vi "backup_imp_test_v9_4.vi"() -> ()   [LabVIEW 2014]
uses:
  <vilib>/eio/EIOPropertyNode/EIOPropertyNode.xnode
  <vilib>/LabVIEW Targets/FPGA/cRIO/shared/nicrio_ModuleControls/nicrio_cRIO-9237_DataRatesRing.ctl
  <vilib>/LabVIEW Targets/FPGA/cRIO/shared/nicrio_ModuleControls/nicrio_cRIO-9237_ExcitationVoltageRing.ctl
  <vilib>/rvi/eio/common/nirviEmuTemplatePropertyGet_errors.vi
  <vilib>/rvi/eio/common/nirviEmuTemplatePropertyGet_noerrors.vi
  <vilib>/rvi/eio/common/nirviEmuTemplatePropertySet_errors.vi
  <vilib>/rvi/eio/common/nirviEmuTemplatePropertySet_noerrors.vi
  <vilib>/eio/EIONode/EIONode.xnode
  <vilib>/rvi/eio/common/nirviEmuTemplateMethod_errors.vi
  <vilib>/rvi/Analysis/measure/butterworth/XNode/niFpgaButterworthFilter.xnode
  <vilib>/rvi/DataTransferAndStorage/Container/XNode/niFpgaContainer.xnode
  <vilib>/rvi/FXPMathLib/FxpSinAndCos/XNode/nifxpmath_SinAndCos.xnode
  <vilib>/rvi/FXPMathLib/FxpSinAndCos/simVIs/DllFxpSinAndCosTemp_sub.vi
  <vilib>/rvi/FXPMathLib/FxpSinAndCos/subVIs/nifxpmath_SinAndCos_SimConfig.ctl
  <vilib>/rvi/interface/RandomDataEmulation/nirviRandomDataFpgaMultiElementTemplate.vi
panel:
  out "omega_y (T) 2":fxp<+/-,36,13>
  out "Dy_d (T) 2":fxp<+/-,36,13>
  out "omega_p (Mavg)":fxp<+/-,36,13>
  out "Dp_d (Mavg)":fxp<+/-,36,13>
  out "omega_p2 (Mavg)":fxp<+/-,36,14>
  out "Dp2_d (Mavg)":fxp<+/-,36,14>
  out "omega_y2 (Mavg)":fxp<+/-,64,27>
  out "Dy2_d (Mavg)":fxp<+/-,36,14>
  in  "mt0_y2":u32
  in  "mt0_p2":u32
  out "Dy_d (Mavg w. f.)":fxp<+/-,36,14>
  out "Dp_d (Mavg w. f.)":fxp<+/-,36,14>
  in  "Dp_d (Mavg) coeff.":i32[](array[numeric])=[946630756, 63555534]
  in  "Dy_d (Mavg) coeff.":i32[](array[numeric])=[946630756, 63555534]
  out "omega_y (Mavg w. f.)":fxp<+/-,36,14>
  in  "omega_y(Mavg) coeff.":i32[](array[numeric])=[946630756, 63555534]
  out "omega_p (Mavg w. f)":fxp<+/-,36,14>
  in  "omega_P(Mavg) coeff.":i32[](array[numeric])=[946630756, 63555534]
  in  "FIFO":i16(ring) items=["Pitch_F+P", "imp ctrl", "Yaw_F+P"]
  out "PID (kHz)":fxp<+/-,20,10>
  in  "Set 6":bool
  in  "Set 5":bool
  in  "Set 4":bool
  in  "Set 3":bool
  in  "Set 2":bool
  in  "Set 1":bool
  out "Dy1_d (T)":fxp<+/-,36,13>
  out "omega_y1 (T)":fxp<+/-,36,13>
  out "Dp1_d (T)":fxp<+/-,36,13>
  out "omega_p1 (T)":fxp<+/-,36,13>
  out "Dy2_d (T)":fxp<+/-,36,13>
  out "Dp2_d (T)":fxp<+/-,36,13>
  out "omega_y2 (T)":fxp<+/-,36,13>
  out "omega_p2 (T)":fxp<+/-,36,13>
  out "mt_omega_y2":u32
  out "mt_omega_p2":u32
  out "rad_y2":fxp<+/-,33,20>
  out "D_y2":fxp<+/-,32,7>
  out "rad_y1":fxp<+/-,33,20>
  out "D_y1":fxp<+/-,32,7>
  out "Encoder Position_y1":i32
  out "Encoder Position_y2":i32
  out "Encoder Position_p2":i32
  out "D_p2":fxp<+/-,32,7>
  out "rad_p2":fxp<+/-,33,20>
  out "D_p1":fxp<+/-,32,7>
  out "rad_p1":fxp<+/-,33,20>
  out "Encoder Position_p1":i32
  in  "Mag. factor_y":fxp<+/-,20,3>
  in  "Mag. encoder_y":bool
  out "omega_y (rad/s)":fxp<+/-,36,13>
  out "Dy_d (mm/s)":fxp<+/-,36,13>
  in  "Vy. Est.":i16(ring) items=["T", "Mavg", "Mavg w. f."]
  out "omega_y1 (Mavg)":fxp<+/-,36,14>
  out "Dy1_d (Mavg)":fxp<+/-,36,14>
  in  "Dy_d_M_avg_Tc (uSec)":i32
  out "Dp1_d (Mavg)":fxp<+/-,36,14>
  out "omega_p1 (Mavg)":fxp<+/-,36,14>
  in  "Dp_d_M_avg_Tc (uSec)":i32
  out "Dp_d (T)":fxp<+/-,36,13>
  out "omega_p (T)":fxp<+/-,36,13>
  in  "Vp. Est.":i16(ring) items=["T", "Mavg", "Mavg w. f."]
  in  "Mag. factor_p":fxp<+/-,20,3>
  in  "Mag. encoder_p":bool
  in  "Belt_out_p":fxp<+/-,7,7>
  in  "Belt_in_p":fxp<+/-,6,6>
  in  "Belt_out_y":fxp<+/-,7,7>
  in  "Belt_in_y":fxp<+/-,6,6>
  out "Fp_dc":fxp<+/-,32,10>
  out "Fy_dc":fxp<+/-,32,10>
  in  "Zero_y":bool
  in  "Zero_p":bool
  in  "mt0_p1":u32
  in  "Encoder reset":bool
  out "fpt_d":fxp<+/-,36,18>
  out "Dp_error_dd":fxp<+/-,36,16>
  out "Dp_error_d":fxp<+/-,33,8>
  in  "Dp_dd coeff.":i32[](array[numeric])=[946630756, 63555534]
  out "Dp_dd":fxp<+/-,36,25>
  out "dFp_PID":fxp<+/-,36,18>
  in  "dFp_PID coeff.":i32[](array[numeric])=[946630756, 63555534]
  out "fpt_i":fxp<+/-,34,18>
  in  "Bv_p":fxp<+/-,22,8>
  in  "Kv_p":fxp<+/-,22,8>
  out "Dp_error":fxp<+/-,22,7>
  out "Dpr_sin":fxp<+/-,22,7>
  in  "Sin offset_p":fxp<+/-,22,7>
  in  "Sin magnitude_p":fxp<+/-,21,6>
  out "Dpr_sin_dd":fxp<+/-,35,20>
  out "Dpr_sin_d":fxp<+/-,33,15>
  out "Sin omega_p":fxp<+/-,34,9>
  in  "Sin wave freq._p (Hz)":fxp<+/-,32,6>
  in  "Dpr_step":fxp<+/-,22,7>
  out "Dpr_for":fxp<+/-,22,7>
  in  "Command_p":i16(ring) items=["Step", "Sine"]
  in  "Ki_p":fxp<+/-,30,9>
  out "Fp_PID":fxp<+/-,36,16>
  in  "fp_tolorance":fxp<+,22,6>
  out "fp_tilde":fxp<+/-,33,10>
  in  "Kd_p":fxp<+/-,30,9>
  in  "Kp_p":fxp<+/-,32,13>
  out "Fr_p":fxp<+/-,32,10>
  in  "S/F coeff_p":fxp<+/-,25,-10>
  in  "S/F coeff_y":fxp<+/-,25,-10>
  out "va_p":fxp<+/-,36,7>
  out "vb_p":fxp<+/-,37,8>
  out "vq_p_F":fxp<+/-,20,5> format="%.57g"
  out "vd_p_F":fxp<+/-,20,5>
  in  "dFp_add":bool
  in  "Stop motor_p":bool
  out "Force_p":fxp<+/-,32,10>
  in  "Strain selection_p":i16(ring) items=["Raw", "Avg.8", "Avg.8 w. filter"]
  out "Strain_p (Avg8 w. f)":fxp<+/-,36,8>
  in  "Strain_p Avg.8 coeff.":i32[](array[numeric])=[946630756, 63555534]
  out "Strain_p (Avg8)":fxp<+/-,36,4>
  out "Raw Strain_p":fxp<+/-,36,4>
  out "Mod6/AI3":fxp<+/-,36,4>
  in  "Strain gage reset_p":bool
  out "Dp_d (mm/s)":fxp<+/-,36,13>
  out "omega_p (rad/s)":fxp<+/-,36,13>
  out "mt_omega_p1":u32
  out "rad_p(NrTheta)":fxp<+/-,33,20>
  out "D_p(mm)":fxp<+/-,32,7>
  out "Encoder Position_p":i32
  in  "Encoder reset_p":bool
  out "Strain_y (Avg8 w. f)":fxp<+/-,36,8>
  in  "Strain_y Avg8 coeff.":i32[](array[numeric])=[-898916953, 1957103773, 3888751]
  out "Dyr_for":fxp<+/-,22,7>
  in  "Command_y":i16(ring) items=["Step", "Sine"]
  out "Strain_y (Avg8)":fxp<+/-,36,4>
  in  "Strain selection_y":i16(ring) items=["Raw", "Avg.8", "Avg.8 w. filter"]
  out "vb_y":fxp<+/-,38,8>
  out "va_y":fxp<+/-,38,8>
  out "fyt_d":fxp<+/-,36,18>
  out "Fr_y":fxp<+/-,32,10>
  in  "Bv_y":fxp<+/-,22,8>
  out "Dy_error_dd":fxp<+/-,36,16>
  out "Dy_error_d":fxp<+/-,33,8>
  in  "Kv_y":fxp<+/-,22,8>
  out "Dy_error":fxp<+/-,22,7>
  out "Dyr_sin_dd":fxp<+/-,35,20>
  out "Dyr_sin_d":fxp<+/-,33,15>
  out "Sin omega_y":fxp<+/-,34,9>
  out "Dyr_sin":fxp<+/-,22,7>
  in  "Sin offset_y":fxp<+/-,22,7>
  in  "Sin magnitude_y":fxp<+/-,21,6>
  out "Time now(s)":fxp<+,52,14>
  in  "Sin wave freq._y (Hz)":fxp<+/-,32,6>
  in  "Dyr_step":fxp<+/-,22,7>
  in  "Drive mode":i16(ring) items=["Backward", "Forward"]
  out "Dy_dd":fxp<+/-,36,25>
  in  "Dy_dd coeff.":i32[](array[numeric])=[946630756, 63555534]
  out "dFy_PID":fxp<+/-,36,18>
  in  "dFy_PID coeff.":i32[](array[numeric])=[946630756, 63555534]
  out "fyt_i":fxp<+/-,36,16>
  out "Fy_PID":fxp<+/-,36,16>
  in  "fy_tolorance":fxp<+,22,6>
  in  "Ki_y":fxp<+/-,30,9>
  in  "Kd_y":fxp<+/-,30,9>
  out "fy_tilde":fxp<+/-,32,10>
  in  "Kp_y":fxp<+/-,32,13>
  out "vq_y_F":fxp<+/-,20,5> format="%.57g"
  out "vd_y_F":fxp<+/-,20,5>
  in  "dFy_add":bool
  in  "Stop motor_y":bool
  out "Dy_d (T)":fxp<+/-,36,13>
  out "omega_y (T)":fxp<+/-,36,13>
  in  "mt0_y1":u32
  out "mt_omega_y1":u32
  out "rad_y(NrTheta)":fxp<+/-,33,20>
  out "D_y(mm)":fxp<+/-,32,7>
  out "Encoder Position_y":i32
  in  "Encoder reset_y":bool
  in  "Ini coe.":bool
  out "Loop rate (kHz)":fxp<+/-,36,7>
  out "Force_y":fxp<+/-,32,10>
  out "Raw Strain_y":fxp<+/-,36,4>
  in  "Strain gage reset_y":bool
  in  "Stop (Strain)":bool
  out "Mod6/AI2":fxp<+/-,36,4>
  in  "Excitation Voltage":T1 items=["2.5 Volts", "3.3 Volts", "5.0 Volts", "10.0 Volts", "External Excitation"]
  in  "Data Rate":T2=1 items=["50.000 kS/s (NI 9237)"=1, "25.000 kS/s (NI 9237)"=2, "16.667 kS/s (NI 9237)"=3, "12.500 kS/s (NI 9237)"=4, "10.000 kS/s (NI 9237)"=5, "8.333 kS/s (NI 9237)"=6, "7.143 kS/s (NI 9237)"=7, "6.250 kS/s (NI 9237)"=8, "5.556 kS/s (NI 9237)"=9, "5.000 kS/s (NI 9237)"=10, "4.545 kS/s (NI 9237)"=11, "4.167 kS/s (NI 9237)"=12, "3.846 kS/s (NI 9237)"=13, "3.571 kS/s (NI 9237)"=14, "3.333 kS/s (NI 9237)"=15, "3.125 kS/s (NI 9237)"=16, "2.941 kS/s (NI 9237)"=17, "2.778 kS/s (NI 9237)"=18, "2.632 kS/s (NI 9237)"=19, "2.500 kS/s (NI 9237)"=20, "2.381 kS/s (NI 9237)"=21, "2.273 kS/s (NI 9237)"=22, "2.174 kS/s (NI 9237)"=23, "2.083 kS/s (NI 9237)"=24, "2.000 kS/s (NI 9237)"=25, "1.923 kS/s (NI 9237)"=26, "1.852 kS/s (NI 9237)"=27, "1.786 kS/s (NI 9237)"=28, "1.724 kS/s (NI 9237)"=29, "1.667 kS/s (NI 9237)"=30, "1.613 kS/s (NI 9237)"=31]
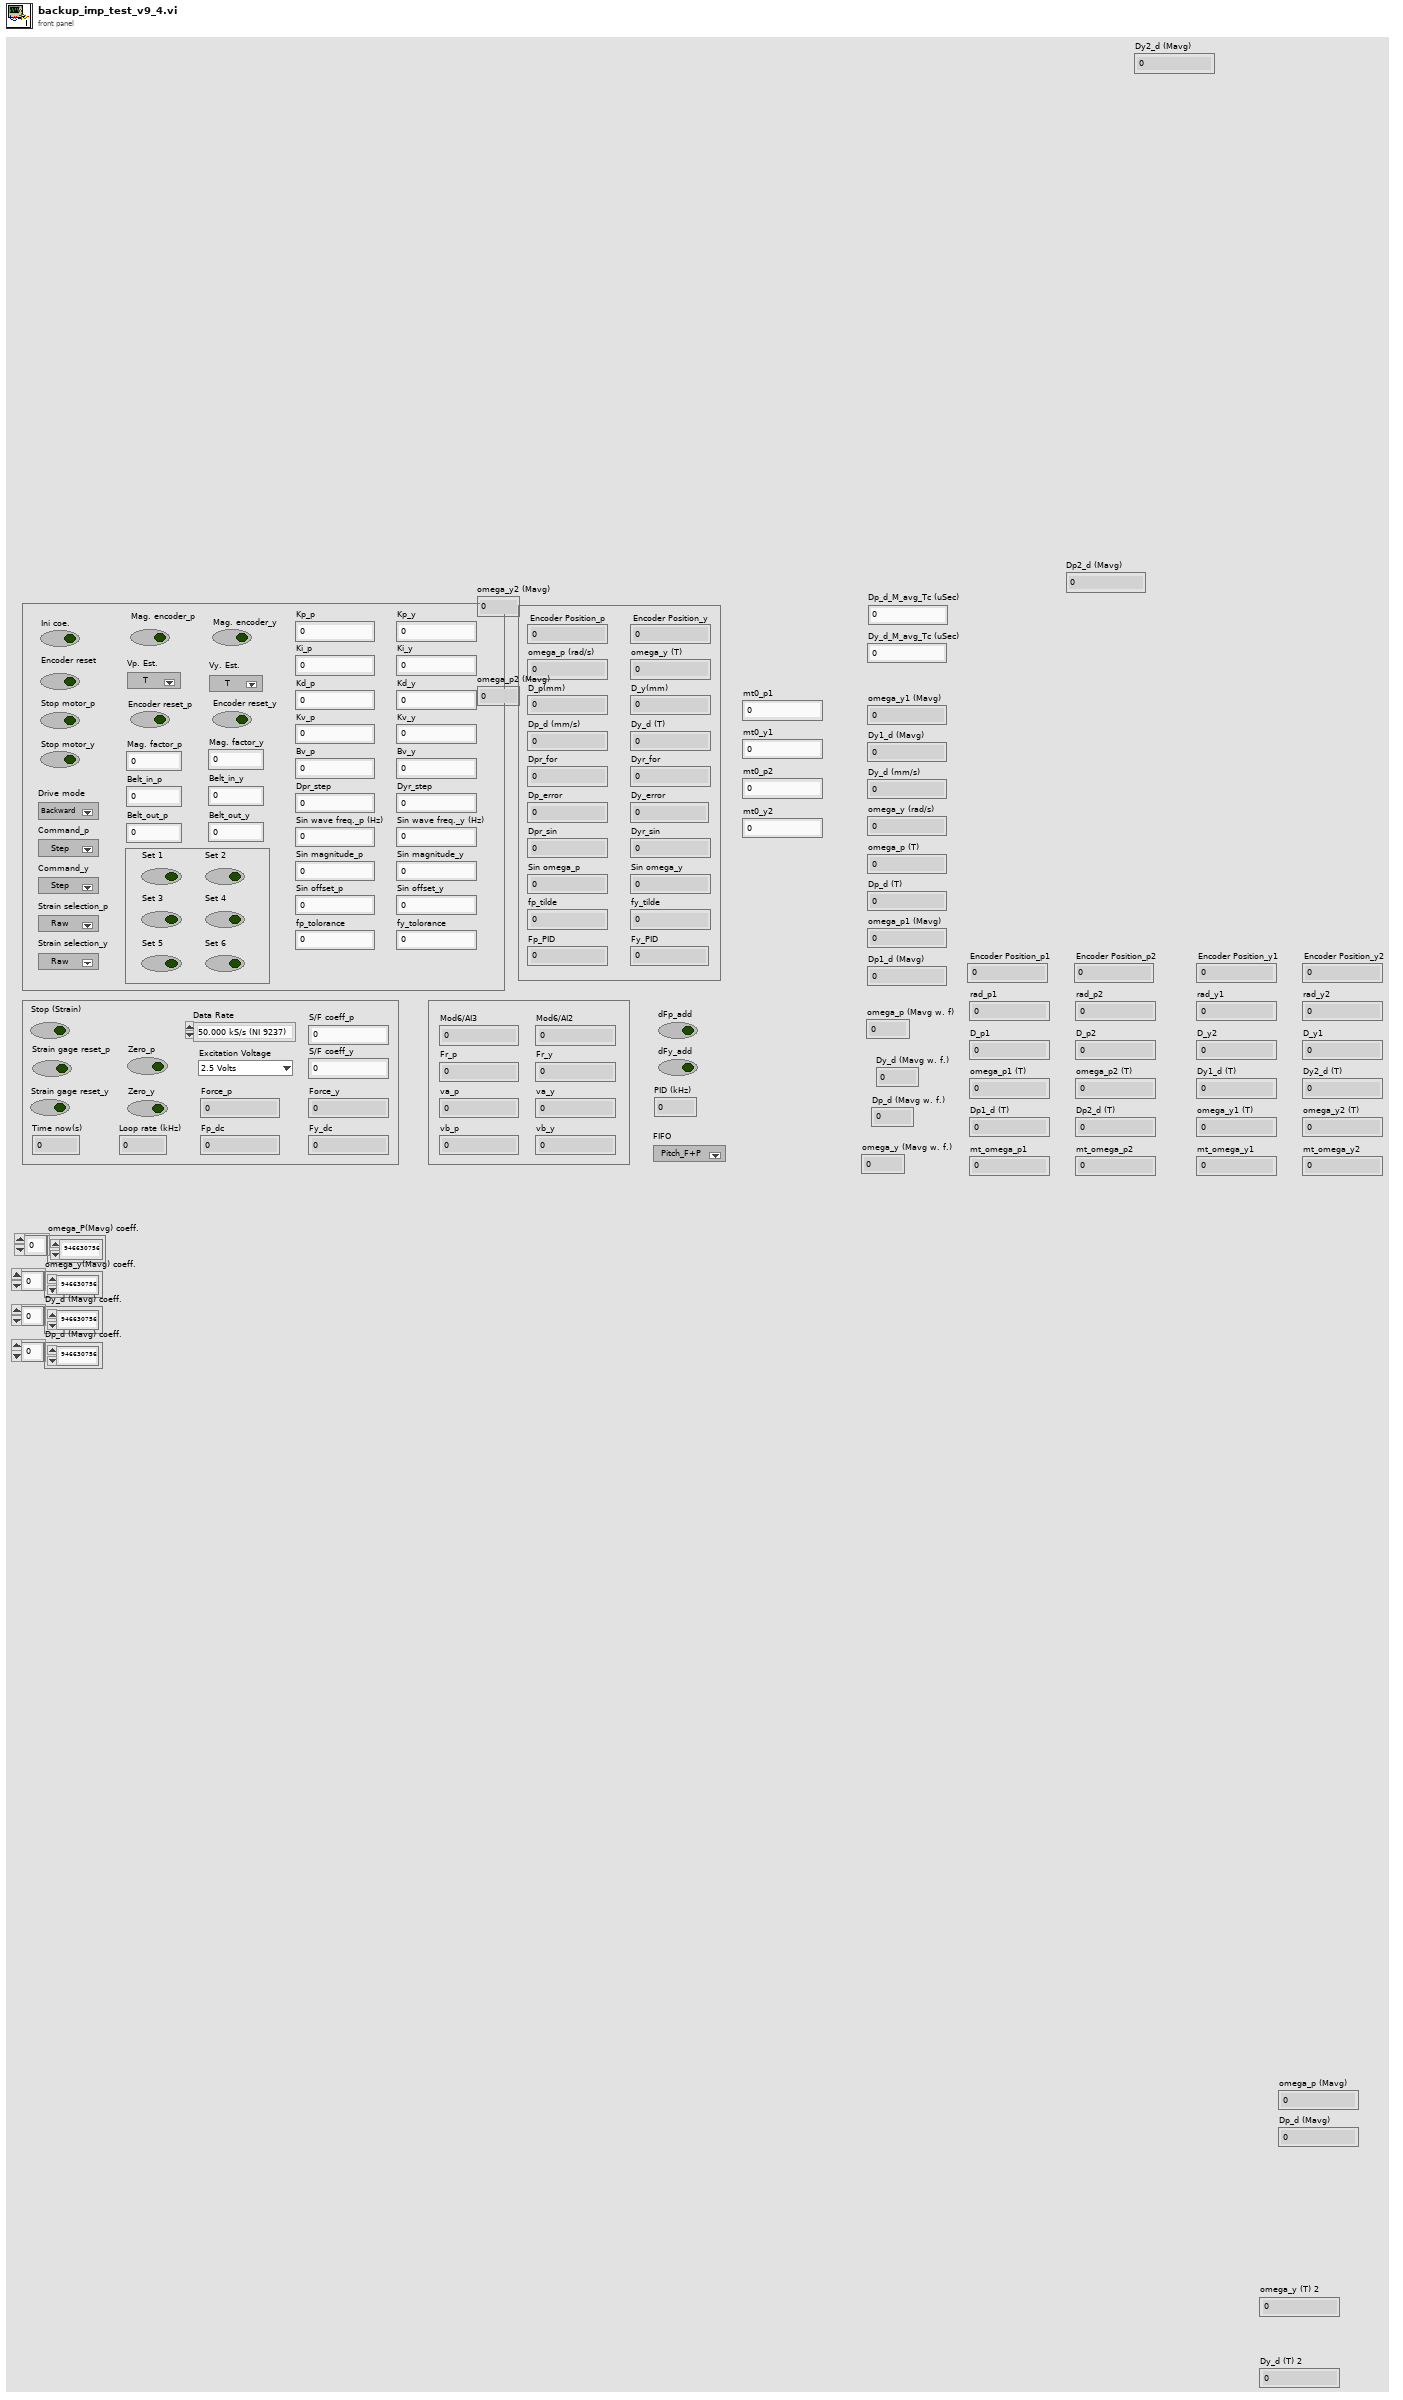
[diagram p1: front panel]
types:
  T1 = typedef "nicrio_cRIO-9237_ExcitationVoltageRing.ctl" = u8
  T2 = typedef "nicrio_cRIO-9237_DataRatesRing.ctl" = u8
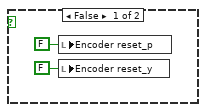
[diagram p12: hidden frame]
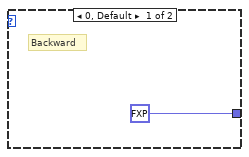
[diagram p13: hidden frame]
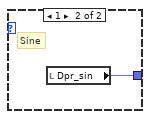
[diagram p14: hidden frame]
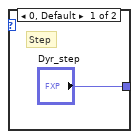
[diagram p15: hidden frame]
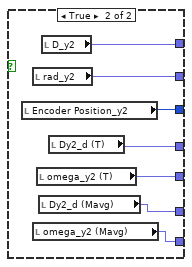
[diagram p16: hidden frame]
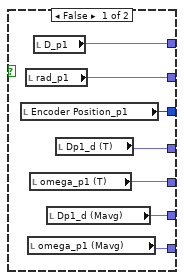
[diagram p17: hidden frame]
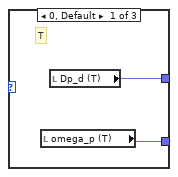
[diagram p18: hidden frame]
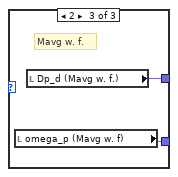
[diagram p19: hidden frame]
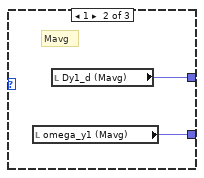
[diagram p20: hidden frame]
diagram:
  w2 = 25
  w5 = i16 25
  w13 = 25
  w16 = 25
  w21 = TRUE ("Half-Bridge Enable")
  # "Encoder 4096ppr\nomega = 61359.2315154/mt\nomega0 = 2*pi/4096 (rad/s)"
  # "Encoder 800ppr\nomega = 314159.265359/mt\nomega0 = 2*pi/800 (rad/s)"
  # "v9\nKp改32/13\nKd改30/9\nKo改30/9"
  # "Resolutuin of Mag. Encoder = 4096*(F_mag)"
  # "use Mavg method to estimate omega or velocity from magnetic encoder"
  # "為什麼要寫兩個迴圈?\nv9後已修正"
  # "Dr_dd ?"
  # "Dr_d ?"
  n1 = xnode "FPGA I/O Property Node"("error in"=errorcluster {"status"=FALSE, "code"=0, "source"=""}, "Data Rate"="Data Rate", "Excitation Voltage"="Excitation Voltage") -> ("error out"=w26:errorcluster)  [unwired: 1 in, 1 out]
  n2 = xnode "FPGA I/O Property Node"("error in"=w26, "Half-Bridge Enable"=w21) -> ("error out"=w19:errorcluster)  [unwired: 1 in, 1 out]
  n3 = xnode "FPGA I/O Property Node"("Half-Bridge Enable"=w21) -> ("error out"=w18:errorcluster)  [unwired: 2 in, 1 out]
  n4 = Merge Errors(w19, w18) -> (w20:errorcluster)
  n5 = xnode "FPGA I/O Node"("error in"=w20, "Mod6/Start"=TRUE) -> ("error out"=w24:errorcluster)  [unwired: 1 in, 1 out]
  n6 = while "AO_p" {
    stop <- FALSE stop-if-true
    n7 = flat-sequence {
      frame #0 {
        n8 = local read "rad_p(NrTheta)"() -> (w41:fxp<+/-,33,20>)
        n9 = local read "vq_p_F"() -> (w42:fxp<+/-,20,5>)
        n10 = local read "vd_p_F"() -> (w44:fxp<+/-,20,5>)
        n11 = Select(t=fxp<+/-,20,5> 0.0, s="Stop motor_p", f=w44) -> (s? t:f=w33:fxp<+/-,20,5>)
        n12 = Select(t=fxp<+,1,1> 0.0, s="Stop motor_p", f=w42) -> (s? t:f=w32:fxp<+/-,20,5>)
        n13 = xnode "High Throughput Sine & Cosine"("x (pi)"=w41) -> ("sin(x)"=w35:fxp<+/-,16,2>, "cos(x)"=w34:fxp<+/-,16,2>)
        n14 = Negate(x=w32) -> (-x=w40:fxp<+/-,21,6>)
        n15 = Multiply(x=w33, y=w35) -> (x*y=w39:fxp<+/-,36,7>)
        n16 = Multiply(x=w33, y=w34) -> (x*y=w37:fxp<+/-,36,7>)
        n17 = Multiply(x=w34, y=w32) -> (x*y=w38:fxp<+/-,36,7>)
        n18 = Multiply(x=w35, y=w40) -> (x*y=w36:fxp<+/-,35,6>)
        n19 = Add(x=w39, y=w38) -> (x+y=→"vb_p":fxp<+/-,37,8>)
        n20 = Add(x=w37, y=w36) -> (x+y=→"va_p":fxp<+/-,36,7>)
      }
      frame #1 {
        n21 = local read "Encoder reset_p"() -> (w77:bool)
        n22 = local read "vb_p"() -> (w78:fxp<+/-,37,8>)
        n23 = local read "va_p"() -> (w79:fxp<+/-,36,7>)
        n24 = Select(t=fxp<+,2,2> 3.0, s=w77, f=w79) -> (s? t:f=w85:fxp<+/-,36,7>)
        n25 = Select(t=fxp<+,1,1> 0.0, s=w77, f=w78) -> (s? t:f=w84:fxp<+/-,37,8>)
        n26 = Multiply(x=w85, y=fxp<+/-,1,0> -0.5) -> (x*y=w80:fxp<+/-,36,6>)
        n27 = Multiply(x=w84, y=fxp<+/-,1,0> -0.5) -> (x*y=w81:fxp<+/-,36,6>)
        n28 = xnode "FPGA I/O Node"("Mod8/AO0"=w80, "Mod8/AO1"=w81) -> ()  [unwired: 2 in, 2 out]
      }
    }
  }
  n29 = while "AO_y" {
    stop <- FALSE stop-if-true
    n30 = flat-sequence {
      frame #0 {
        n31 = local read "rad_y(NrTheta)"() -> (w105:fxp<+/-,33,20>)
        n32 = local read "vd_y_F"() -> (w103:fxp<+/-,20,5>)
        n33 = local read "vq_y_F"() -> (w102:fxp<+/-,20,5>)
        n34 = Select(t=fxp<+/-,20,5> 0.0, s="Stop motor_y", f=w103) -> (s? t:f=w97:fxp<+/-,20,5>)
        n35 = Select(t=fxp<+/-,20,5> 0.0, s="Stop motor_y", f=w102) -> (s? t:f=w96:fxp<+/-,20,5>)
        n36 = xnode "High Throughput Sine & Cosine"("x (pi)"=w105) -> ("sin(x)"=w99:fxp<+/-,17,2>, "cos(x)"=w98:fxp<+/-,17,2>)
        n37 = Negate(x=w96) -> (-x=w95:fxp<+/-,21,6>)
        n38 = Multiply(x=w97, y=w99) -> (x*y=w94:fxp<+/-,37,7>)
        n39 = Multiply(x=w97, y=w98) -> (x*y=w92:fxp<+/-,37,7>)
        n40 = Multiply(x=w98, y=w96) -> (x*y=w93:fxp<+/-,37,7>)
        n41 = Multiply(x=w99, y=w95) -> (x*y=w91:fxp<+/-,36,6>)
        n42 = Add(x=w94, y=w93) -> (x+y=→"vb_y":fxp<+/-,38,8>)
        n43 = Add(x=w92, y=w91) -> (x+y=→"va_y":fxp<+/-,37,7>)
      }
      frame #1 {
        n44 = local read "Encoder reset_y"() -> (w138:bool)
        n45 = local read "va_y"() -> (w137:fxp<+/-,38,8>)
        n46 = local read "vb_y"() -> (w136:fxp<+/-,38,8>)
        n47 = Select(t=fxp<+,2,2> 3.0, s=w138, f=w137) -> (s? t:f=w142:fxp<+/-,38,8>)
        n48 = Select(t=fxp<+,1,1> 0.0, s=w138, f=w136) -> (s? t:f=w141:fxp<+/-,38,8>)
        n49 = Multiply(x=w142, y=fxp<+/-,1,0> -0.5) -> (x*y=w145:fxp<+/-,39,8>)
        n50 = Multiply(x=w141, y=fxp<+/-,1,0> -0.5) -> (x*y=w146:fxp<+/-,37,6>)
        n51 = xnode "FPGA I/O Node"("Mod8/AO2"=w145, "Mod8/AO3"=w146) -> ()  [unwired: 2 in, 2 out]
      }
    }
  }
  n52 = while "Selection" {
    stop <- FALSE stop-if-true
    # "T = Mag. encoder\nF = Motor encoder"
    n53 = case shown="2" "Strain selection_y" {
      tunnel: [w229 w230 w231] -> w182
      frame 0, Default {
        n54 = local read "Raw Strain_y"() -> (w229:fxp<+/-,36,4>)
      }
      frame 1 {
        n55 = local read "Strain_y (Avg8)"() -> (w230:fxp<+/-,36,4>)
      }
      frame 2 {
        n56 = local read "Strain_y (Avg8 w. f)"() -> (w231:fxp<+/-,36,8>)
      }
    }
    n57 = case shown="1" "Vp. Est." {
      tunnel: [w213 w214 w217] -> w165
      tunnel: [w212 w215 w216] -> w166
      frame 0, Default {
        # "T"
        n58 = local read "omega_p (T)"() -> (w213:fxp<+/-,36,13>)
        n59 = local read "Dp_d (T)"() -> (w212:fxp<+/-,36,13>)
      }
      frame 1 {
        # "Mavg"
        n60 = local read "omega_p1 (Mavg)"() -> (w214:fxp<+/-,36,14>)
        n61 = local read "Dp1_d (Mavg)"() -> (w215:fxp<+/-,36,14>)
      }
      frame 2 {
        # "Mavg w. f."
        n62 = local read "omega_p (Mavg w. f)"() -> (w217:fxp<+/-,36,14>)
        n63 = local read "Dp_d (Mavg w. f.)"() -> (w216:fxp<+/-,36,14>)
      }
    }
    "Dp_d (mm/s)" <- w166
    "omega_p (rad/s)" <- w165
    n64 = Divide(x=w182, y="S/F coeff_y") -> (x/y=w175:fxp<+/-,32,10>)
    n65 = case shown="True" "Zero_y" {
      tunnel: w175 -> [_ w225]
      frame False {
      }
      frame True {
        "Fy_dc" <- w225
      }
    }
    n66 = local read "Fy_dc"() -> (w176:fxp<+/-,32,10>)
    n67 = Subtract(x=w175, y=w176) -> (x-y=→"Force_y":fxp<+/-,33,11>)
    n68 = case shown="2" "Strain selection_p" {
      tunnel: [w226 w227 w228] -> w180
      frame 0, Default {
        n69 = local read "Raw Strain_p"() -> (w226:fxp<+/-,36,4>)
      }
      frame 1 {
        n70 = local read "Strain_p (Avg8)"() -> (w227:fxp<+/-,36,4>)
      }
      frame 2 {
        n71 = local read "Strain_p (Avg8 w. f)"() -> (w228:fxp<+/-,36,8>)
      }
    }
    n72 = case shown="0, Default" "Vy. Est." {
      tunnel: [w219 w221 w223] -> w168
      tunnel: [w218 w220 w222] -> w169
      frame 0, Default {
        # "T"
        n73 = local read "omega_y (T)"() -> (w218:fxp<+/-,36,13>)
        n74 = local read "Dy_d (T)"() -> (w219:fxp<+/-,36,13>)
      }
      frame 1 {
        # "Mavg"
        n75 = local read "omega_y1 (Mavg)"() -> (w220:fxp<+/-,36,14>)
        n76 = local read "Dy1_d (Mavg)"() -> (w221:fxp<+/-,36,14>)
      }
      frame 2 {
        # "Mavg w. f."
        n77 = local read "omega_y (Mavg w. f.)"() -> (w222:fxp<+/-,36,14>)
        n78 = local read "Dy_d (Mavg w. f.)"() -> (w223:fxp<+/-,36,14>)
      }
    }
    "Dy_d (mm/s)" <- w168
    "omega_y (rad/s)" <- w169
    n79 = Divide(x=w180, y="S/F coeff_p") -> (x/y=w172:fxp<+/-,32,10>)
    n80 = case shown="True" "Zero_p" {
      tunnel: w172 -> [_ w224]
      frame False {
      }
      frame True {
        "Fp_dc" <- w224
      }
    }
    n81 = local read "Fp_dc"() -> (w170:fxp<+/-,32,10>)
    n82 = Subtract(x=w172, y=w170) -> (x-y=→"Force_p":fxp<+/-,33,11>)
    n83 = case shown="False" "Mag. encoder_y" {
      tunnel: [w190 w196] -> w156
      tunnel: [w189 w197] -> w157
      tunnel: [w188 w195] -> w159
      tunnel: [w186 w194] -> w153
      tunnel: [w187 w193] -> w152
      tunnel: [w185 w192] -> w148
      tunnel: [w184 w191] -> w147
      frame False {
        n84 = local read "Encoder Position_y1"() -> (w188:i32)
        n85 = local read "omega_y1 (Mavg)"() -> (w184:fxp<+/-,36,14>)
        n86 = local read "Dy1_d (Mavg)"() -> (w185:fxp<+/-,36,14>)
        n87 = local read "rad_y1"() -> (w190:fxp<+/-,33,20>)
        n88 = local read "omega_y1 (T)"() -> (w186:fxp<+/-,36,13>)
        n89 = local read "D_y1"() -> (w189:fxp<+/-,32,7>)
        n90 = local read "Dy1_d (T)"() -> (w187:fxp<+/-,36,13>)
      }
      frame True {
        n91 = local read "Encoder Position_y2"() -> (w195:i32)
        n92 = local read "rad_y2"() -> (w196:fxp<+/-,33,20>)
        n93 = local read "omega_y2 (Mavg)"() -> (w191:fxp<+/-,64,27>)
        n94 = local read "omega_y2 (T)"() -> (w194:fxp<+/-,36,13>)
        n95 = local read "Dy2_d (Mavg)"() -> (w192:fxp<+/-,36,14>)
        n96 = local read "D_y2"() -> (w197:fxp<+/-,32,7>)
        n97 = local read "Dy2_d (T)"() -> (w193:fxp<+/-,36,13>)
      }
    }
    "D_y(mm)" <- w157
    "rad_y(NrTheta)" <- w156
    "Encoder Position_y" <- w159
    "Dy_d (T)" <- w152
    "omega_y (T)" <- w153
    "Dy_d (T) 2" <- w148
    "omega_y (T) 2" <- w147
    n98 = case shown="True" "Mag. encoder_p" {
      tunnel: [w204 w211] -> w161
      tunnel: [w203 w210] -> w162
      tunnel: [w202 w209] -> w163
      tunnel: [w200 w208] -> w155
      tunnel: [w201 w207] -> w154
      tunnel: [w199 w205] -> w151
      tunnel: [w198 w206] -> w150
      frame False {
        n99 = local read "Encoder Position_p1"() -> (w202:i32)
        n100 = local read "rad_p1"() -> (w203:fxp<+/-,33,20>)
        n101 = local read "omega_p1 (Mavg)"() -> (w198:fxp<+/-,36,14>)
        n102 = local read "omega_p1 (T)"() -> (w200:fxp<+/-,36,13>)
        n103 = local read "D_p1"() -> (w204:fxp<+/-,32,7>)
        n104 = local read "Dp1_d (Mavg)"() -> (w199:fxp<+/-,36,14>)
        n105 = local read "Dp1_d (T)"() -> (w201:fxp<+/-,36,13>)
      }
      frame True {
        n106 = local read "Encoder Position_p2"() -> (w209:i32)
        n107 = local read "omega_p2 (Mavg)"() -> (w206:fxp<+/-,36,14>)
        n108 = local read "rad_p2"() -> (w210:fxp<+/-,33,20>)
        n109 = local read "D_p2"() -> (w211:fxp<+/-,32,7>)
        n110 = local read "Dp2_d (Mavg)"() -> (w205:fxp<+/-,36,14>)
        n111 = local read "omega_p2 (T)"() -> (w208:fxp<+/-,36,13>)
        n112 = local read "Dp2_d (T)"() -> (w207:fxp<+/-,36,13>)
      }
    }
    "D_p(mm)" <- w161
    "rad_p(NrTheta)" <- w162
    "Encoder Position_p" <- w163
    "Dp_d (T)" <- w154
    "omega_p (T)" <- w155
    "Dp_d (Mavg)" <- w151
    "omega_p (Mavg)" <- w150
  }
  n113 = while "Quadrature drive_y" {
    stop <- FALSE stop-if-true
    n114 = local read "dFy_PID"() -> (w233:fxp<+/-,36,18>)
    n115 = local read "omega_y (rad/s)"() -> (w241:fxp<+/-,36,13>)
    n116 = local read "Fy_PID"() -> (w234:fxp<+/-,36,16>)
    n117 = Select(t=w233, s="dFy_add", f=fxp<+,1,1> 0.0) -> (s? t:f=w237:fxp<+/-,36,18>)
    n118 = call "Oriental_step_motor_PKP225.vi"("F_Threshold"=fxp<+,12,12> 10.0, "dFmr"=w237, "omega"=w241, "Fmr"=w234) -> ("vq_F"=→"vq_y_F":fxp<+/-,20,5>, "vd_F"=→"vd_y_F":fxp<+/-,20,5>)  [unwired: 6 in]
  }
  n119 = while "Encoder_p" {
    shift-right: [w279] -> _
    shift-left: _ -> [w278]
    shift-right: [w280] -> _
    shift-left: _ -> [w277]
    shift-right: [w274] -> _
    shift-left: _ -> [w276]
    shift-right: [w265] -> _
    shift-left: _ -> [w264]
    shift-right: [w266] -> _
    shift-left: _ -> [w267]
    shift-right: [w261] -> _
    shift-left: _ -> [w262]
    stop <- FALSE stop-if-true
    w257 = fxp<+/-,20,-5> 0.00048828125  # L/4096
    w255 = fxp<+/-,16,1> 0.0244140625  # 2*50/4096
    w273 = fxp<+/-,20,-5> 0.002499997615814209  # L/800
    w247 = fxp<+/-,16,1> 0.125  # 2*50/800
    n120 = xnode "FPGA I/O Node"() -> ("Mod7/DIO0"=w282:bool, "Mod7/DIO1"=w281:bool)  [unwired: 2 in, 2 out]
    n121 = xnode "FPGA I/O Node"() -> ("Mod7/DIO4"=w269:bool, "Mod7/DIO5"=w268:bool)  [unwired: 2 in, 2 out]
    n122 = local read "Encoder reset_p"() -> (w263:bool)
    n123 = call "encoder_sub.vi"("A_pre"=w278, "B_pre"=w277, "Encoder Position_pre"=w276, "A input"=w282, "Encoder Position Reset"="Encoder reset_p", "B input"=w281) -> ("A"=w279:bool, "B"=w280:bool, "Encoder Position (Counts)"=w274:i32)  [unwired: 19 in]
    "Encoder Position_p1" <- w274
    n124 = call "encoder_sub.vi"("A_pre"=w264, "B_pre"=w267, "Encoder Position_pre"=w262, "A input"=w269, "Encoder Position Reset"=w263, "B input"=w268) -> ("A"=w265:bool, "B"=w266:bool, "Encoder Position (Counts)"=w261:i32)  [unwired: 19 in]
    "Encoder Position_p2" <- w261
    n125 = local read "Belt_in_p"() -> (w272:fxp<+/-,6,6>)
    n126 = local read "Belt_in_p"() -> (w258:fxp<+/-,6,6>)
    n127 = local read "Belt_out_p"() -> (w270:fxp<+/-,7,7>)
    n128 = To Fixed-Point(number=w261) -> (fixed-point=w243:fxp<+/-,32,32>)  [unwired: 1 in]
    n129 = To Fixed-Point(number=w274) -> (fixed-point=w248:fxp<+/-,32,32>)  [unwired: 1 in]
    n130 = local read "Belt_out_p"() -> (w260:fxp<+/-,7,7>)
    n131 = local read "Mag. factor_p"() -> (w254:fxp<+/-,20,3>)
    n132 = Divide(x=w257, y="Mag. factor_p") -> (x/y=w256:fxp<+/-,41,13>)
    n133 = Multiply(x=w273, y=w272) -> (x*y=w271:fxp<+/-,26,1>)
    n134 = Multiply(x=w256, y=w258) -> (x*y=w259:fxp<+/-,46,18>)
    n135 = Divide(x=w271, y=w270) -> (x/y=w250:fxp<+/-,33,1>)
    n136 = Divide(x=w259, y=w260) -> (x/y=w245:fxp<+/-,53,18>)
    n137 = Divide(x=w255, y=w254) -> (x/y=w242:fxp<+/-,32,1>)
    n138 = Multiply(x=w248, y=w247) -> (x*y=→"rad_p1":fxp<+/-,33,20>)
    n139 = Multiply(x=w245, y=w243) -> (x*y=→"D_p2":fxp<+/-,37,7>)
    n140 = Multiply(x=w243, y=w242) -> (x*y=→"rad_p2":fxp<+/-,33,20>)
    n141 = Multiply(x=w250, y=w248) -> (x*y=→"D_p1":fxp<+/-,32,7>)
  }
  n142 = while "Integral and derivative" {
    shift-right: [w338] -> _
    shift-left: _ -> [w337]
    shift-right: [w330] -> _
    shift-left: _ -> [w329]
    shift-right: [w340] -> _
    shift-left: _ -> [w341]
    shift-right: [w320] -> _
    shift-left: _ -> [w319]
    shift-right: [w306] -> _
    shift-left: _ -> [w309]
    shift-right: [w299] -> _
    shift-left: _ -> [w298]
    shift-right: [w293] -> _
    shift-left: _ -> [w292]
    shift-right: [w288] -> _
    shift-left: _ -> [w289]
    stop <- FALSE stop-if-true
    # "Pitch"
    # "Yaw"
    n143 = local read "Dp_d (mm/s)"() -> (w288:fxp<+/-,36,13>)
    n144 = local read "Dy_d (mm/s)"() -> (w320:fxp<+/-,36,13>)
    n145 = local read "Fp_PID"() -> (w293:fxp<+/-,36,16>)
    n146 = local read "fp_tilde"() -> (w310:fxp<+/-,33,10>)
    n147 = local read "fp_tolorance"() -> (w313:fxp<+,22,6>)
    n148 = local read "fy_tolorance"() -> (w316:fxp<+,22,6>)
    n149 = local read "fy_tilde"() -> (w342:fxp<+/-,32,10>)
    n150 = local read "Fy_PID"() -> (w340:fxp<+/-,36,16>)
    n151 = Subtract(x=w293, y=w292) -> (x-y=w297:fxp<+/-,37,17>)
    n152 = Subtract(x=w288, y=w289) -> (x-y=w290:fxp<+/-,37,14>)
    n153 = Absolute Value(x=w310) -> (abs(x)=w314:fxp<+,33,10>)
    n154 = Absolute Value(x=w342) -> (abs(x)=w344:fxp<+,32,10>)
    n155 = Subtract(x=w340, y=w341) -> (x-y=w328:fxp<+/-,37,17>)
    n156 = Subtract(x=w320, y=w319) -> (x-y=w322:fxp<+/-,36,11>)
    n157 = Greater?(x=w344, y=w316) -> (0:w345:bool)
    n158 = Greater?(x=w314, y=w313) -> (0:w312:bool)
    n159 = Multiply(x=fxp<+,7,10> 1000.0, y=w297) -> (x*y=w295:fxp<+/-,32,18>)
    n160 = Multiply(x=fxp<+,7,10> 1000.0, y=w290) -> (x*y=w286:fxp<+/-,36,21>)
    n161 = local read "Stop motor_y"() -> (w331:bool)
    n162 = local read "Stop motor_p"() -> (w301:bool)
    n163 = Select(t=w342, s=w345, f=fxp<+/-,33,11> 0.0) -> (s? t:f=w338:fxp<+/-,33,11>)
    n164 = Select(t=w310, s=w312, f=fxp<+,1,1> 0.0) -> (s? t:f=w306:fxp<+/-,33,10>)
    n165 = Multiply(x=fxp<+,7,10> 1000.0, y=w322) -> (x*y=w321:fxp<+/-,36,21>)
    n166 = xnode "Butterworth Filter"("input data"=w295, "scaled coefficients"="dFp_PID coeff.") -> ("output data"=→"dFp_PID":fxp<+/-,36,22>)  [unwired: 1 in]
    n167 = xnode "Butterworth Filter"("input data"=w286, "scaled coefficients"="Dp_dd coeff.") -> ("output data"=→"Dp_dd":fxp<+/-,36,25>)  [unwired: 1 in]
    n168 = Multiply(x=fxp<+,7,10> 1000.0, y=w328) -> (x*y=w325:fxp<+/-,32,18>)
    n169 = Add(x=w337, y=w338) -> (x+y=w343:fxp<+/-,34,12>)
    n170 = Multiply(x=w309, y=w306) -> (x*y=w308:fxp<+/-,34,12>)
    n171 = xnode "Butterworth Filter"("input data"=w321, "scaled coefficients"="Dy_dd coeff.") -> ("output data"=→"Dy_dd":fxp<+/-,36,25>)  [unwired: 1 in]
    n172 = Multiply(x=fxp<+/-,30,12> 0.000499725341796875, y=w343) -> (x*y=w336:fxp<+/-,34,10>)
    n173 = Multiply(x=fxp<+/-,30,12> 0.000499725341796875, y=w308) -> (x*y=w305:fxp<+/-,34,10>)
    n174 = xnode "Butterworth Filter"("input data"=w325, "scaled coefficients"="dFy_PID coeff.") -> ("output data"=→"dFy_PID":fxp<+/-,36,22>)  [unwired: 1 in]
    n175 = Select(t=fxp<+,1,1> 0.0, s=w331, f=fxp<+,1,1> 1.0) -> (s? t:f=w334:fxp<+,1,1>)
    n176 = Select(t=fxp<+,1,1> 0.0, s=w301, f=fxp<+,1,1> 1.0) -> (s? t:f=w303:fxp<+,1,1>)
    n177 = Add(x=w336, y=w329) -> (x+y=w335:fxp<+/-,36,16>)
    n178 = Add(x=w305, y=w298) -> (x+y=w304:fxp<+/-,36,16>)
    n179 = Multiply(x=w335, y=w334) -> (x*y=w330:fxp<+/-,34,18>)
    "fyt_i" <- w330
    n180 = Multiply(x=w304, y=w303) -> (x*y=w299:fxp<+/-,34,18>)
    "fpt_i" <- w299
    n181 = call "Wait"("Count(uSec)"=u32 1000) -> ()  [unwired: 1 out]
  }
  n182 = while {
    stop <- FALSE stop-if-true
    n183 = case shown="True" "Set 3" {
      frame False {
      }
      frame True {
        n184 = local write "fp_tolorance"(fxp<+,22,6> 3.0 ("fp_tolorance")) -> ()
        n185 = local write "Kp_p"(fxp<+/-,36,9> 100.0 ("Kp_p")) -> ()
      }
    }
    n186 = case shown="True" "Set 2" {
      frame False {
      }
      frame True {
        n187 = local write "fp_tolorance"(fxp<+,22,6> 1.5 ("fp_tolorance")) -> ()
        n188 = local write "Kp_p"(fxp<+/-,36,9> 50.0 ("Kp_p")) -> ()
      }
    }
    n189 = case shown="True" "Set 1" {
      frame False {
      }
      frame True {
        n190 = local write "fp_tolorance"(fxp<+,22,6> 3.0 ("fp_tolorance")) -> ()
        n191 = local write "Kp_p"(fxp<+/-,36,9> 50.0 ("Kp_p")) -> ()
      }
    }
    n192 = case shown="True" "Set 5" {
      frame False {
      }
      frame True {
        n193 = local write "fp_tolorance"(fxp<+,22,6> 3.0 ("fp_tolorance")) -> ()
        n194 = local write "Kp_p"(fxp<+/-,36,9> 150.0 ("Kp_p")) -> ()
      }
    }
    n195 = case shown="True" "Set 6" {
      frame False {
      }
      frame True {
        n196 = local write "fp_tolorance"(fxp<+,22,6> 1.5 ("fp_tolorance")) -> ()
        n197 = local write "Kp_p"(fxp<+/-,36,9> 150.0 ("Kp_p")) -> ()
      }
    }
    n198 = case shown="True" "Set 4" {
      frame False {
      }
      frame True {
        n199 = local write "fp_tolorance"(fxp<+,22,6> 1.5 ("fp_tolorance")) -> ()
        n200 = local write "Kp_p"(fxp<+/-,36,9> 100.0 ("Kp_p")) -> ()
      }
    }
  }
  n201 = while "Omega_p(T method)" {
    shift-right: [w429] -> _
    shift-left: _ -> [w427]
    shift-right: [w410] -> _
    shift-left: _ -> [w428]
    shift-right: [w425] -> _
    shift-left: _ -> [w426]
    shift-right: [w403] -> _
    shift-left: _ -> [w402]
    shift-right: [w398] -> _
    shift-left: _ -> [w400]
    shift-right: [w406] -> _
    shift-left: _ -> [w405]
    stop <- FALSE stop-if-true
    w417 = fxp<+/-,32,0> 0.3183098859153688  # L/2/pi
    w422 = fxp<+/-,32,0> 0.3183098859153688  # L/2/pi
    n202 = local read "Encoder Position_p1"() -> (w429:i32)
    n203 = local read "Encoder Position_p2"() -> (w403:i32)
    n204 = call "Tick Count4"() -> ("Tick Count(Ticks)"=w404:u32)
    n205 = call "omega_sub_Encoder_800ppr.vi"("mt0"="mt0_p1", "omega_pre"=w428, "ticks_m_pre"=w426, "ticks"=w404, "count_pre"=w427, "count"=w429) -> ("ticks_m"=w425:u32, "mt"=→"mt_omega_p1":u32, "omega"=w410:fxp<+/-,36,13>)  [unwired: 3 in]
    "omega_p1 (T)" <- w410
    n206 = call "omega_sub_Encoder_4096ppr.vi"("mt0"="mt0_p2", "omega_pre"=w400, "ticks_m_pre"=w405, "ticks"=w404, "count_pre"=w402, "count"=w403) -> ("ticks_m"=w406:u32, "mt"=→"mt_omega_p2":u32, "omega"=w398:fxp<+/-,20,9>)  [unwired: 3 in]
    n207 = local read "Mag. factor_p"() -> (w418:fxp<+/-,20,3>)
    n208 = local read "Belt_in_p"() -> (w415:fxp<+/-,6,6>)
    n209 = local read "Belt_out_p"() -> (w414:fxp<+/-,7,7>)
    n210 = Multiply(x=w422, y="Belt_in_p") -> (x*y=w420:fxp<+/-,38,6>)
    n211 = Multiply(x=w417, y=w415) -> (x*y=w416:fxp<+/-,38,6>)
    n212 = Divide(x=w420, y="Belt_out_p") -> (x/y=w411:fxp<+/-,20,1>)
    n213 = Divide(x=w398, y=w418) -> (x/y=w399:fxp<+/-,32,1>)
    "omega_p2 (T)" <- w399
    n214 = Divide(x=w416, y=w414) -> (x/y=w409:fxp<+/-,45,6>)
    n215 = Multiply(x=w409, y=w399) -> (x*y=→"Dp2_d (T)":fxp<+/-,36,13>)
    n216 = Multiply(x=w411, y=w410) -> (x*y=→"Dp1_d (T)":fxp<+/-,36,13>)
  }
  n217 = while "PD position controller_y" {
    stop <- FALSE stop-if-true
    n218 = case shown="0, Default" "Drive mode" {
      tunnel: [fxp<+/-,62,19> 0.0 w435] -> w431
      frame 0, Default {
        # "Backward"
      }
      frame 1 {
        # "Forward"
        n219 = local read "Dy_error_d"() -> (w437:fxp<+/-,33,8>)
        n220 = local read "D_y(mm)"() -> (w442:fxp<+/-,32,7>)
        n221 = local read "Dyr_for"() -> (w434:fxp<+/-,22,7>)
        n222 = Subtract(x=w434, y=w442) -> (x-y=w441:fxp<+/-,33,8>)
        "Dy_error" <- w441
        n223 = Multiply(x=w441, y="Kv_y") -> (x*y=w439:fxp<+/-,54,15>)
        n224 = Multiply(x=w437, y="Bv_y") -> (x*y=w436:fxp<+/-,55,16>)
        n225 = Add(x=w439, y=w436) -> (x+y=w435:fxp<+/-,55,16>)
      }
    }
    "Fr_y" <- w431
  }
  n226 = while "Command type" {
    stop <- FALSE stop-if-true
    n227 = case shown="1" "Command_y" {
      tunnel: ["Dyr_step" w451] -> w446
      frame 0, Default {
        # "Step"
      }
      frame 1 {
        # "Sine"
        n228 = local read "Dyr_sin"() -> (w451:fxp<+/-,22,7>)
      }
    }
    "Dyr_for" <- w446
    n229 = case shown="0, Default" "Command_p" {
      tunnel: ["Dpr_step" w449] -> w444
      frame 0, Default {
        # "Step"
      }
      frame 1 {
        # "Sine"
        n230 = local read "Dpr_sin"() -> (w449:fxp<+/-,22,7>)
      }
    }
    "Dpr_for" <- w444
  }
  n231 = while "Sine wave gene" {
    stop <- FALSE stop-if-true
    w457 = fxp<+,20,3> 6.2831878662109375  # 2*pi
    w489 = fxp<+,20,3> 6.2831878662109375  # 2*pi
    n232 = local read "Time now(s)"() -> (w495:fxp<+,52,14>)
    n233 = local read "Sin wave freq._y (Hz)"() -> (w488:fxp<+/-,32,6>)
    n234 = Multiply(x="Sin wave freq._y (Hz)", y=fxp<+/-,10,3> 2.0) -> (x*y=w496:fxp<+/-,41,9>)
    n235 = local read "Sin magnitude_y"() -> (w486:fxp<+/-,21,6>)
    n236 = local read "Sin magnitude_y"() -> (w479:fxp<+/-,21,6>)
    n237 = local read "Sin omega_y"() -> (w482:fxp<+/-,34,9>)
    n238 = Multiply(x=w496, y=w495) -> (x*y=w494:fxp<+/-,41,19>)
    n239 = Square(x=w482) -> (x^2=w481:fxp<+,34,18>)
    n240 = xnode "High Throughput Sine & Cosine"("x (pi)"=w494) -> ("sin(x)"=w476:fxp<+/-,16,2>, "cos(x)"=w484:fxp<+/-,16,2>)
    n241 = Multiply(x=w489, y=w488) -> (x*y=w487:fxp<+/-,34,9>)
    "Sin omega_y" <- w487
    n242 = Negate(x=w481) -> (-x=w480:fxp<+/-,35,19>)
    n243 = Multiply(x=w487, y=w486) -> (x*y=w485:fxp<+/-,33,15>)
    n244 = Multiply(x=w480, y=w479) -> (x*y=w478:fxp<+/-,34,20>)
    n245 = Multiply(x=w484, y=w485) -> (x*y=→"Dyr_sin_d":fxp<+/-,33,15>)
    n246 = Multiply(x="Sin magnitude_y", y=w476) -> (x*y=w492:fxp<+/-,37,8>)
    n247 = Multiply(x=w476, y=w478) -> (x*y=→"Dyr_sin_dd":fxp<+/-,35,20>)
    n248 = Add(x=w492, y="Sin offset_y") -> (x+y=→"Dyr_sin":fxp<+/-,37,8>)
    n249 = local read "Sin wave freq._p (Hz)"() -> (w453:fxp<+/-,32,6>)
    n250 = local read "Time now(s)"() -> (w471:fxp<+,52,14>)
    n251 = local read "Sin magnitude_p"() -> (w454:fxp<+/-,21,6>)
    n252 = local read "Sin magnitude_p"() -> (w456:fxp<+/-,21,6>)
    n253 = local read "Sin omega_p"() -> (w455:fxp<+/-,34,9>)
    n254 = Multiply(x="Sin wave freq._p (Hz)", y=fxp<+/-,10,3> 2.0) -> (x*y=w475:fxp<+/-,42,9>)
    n255 = Multiply(x=w475, y=w471) -> (x*y=w472:fxp<+/-,41,19>)
    n256 = Square(x=w455) -> (x^2=w467:fxp<+,34,18>)
    n257 = xnode "High Throughput Sine & Cosine"("x (pi)"=w472) -> ("sin(x)"=w458:fxp<+/-,16,2>, "cos(x)"=w463:fxp<+/-,16,2>)
    n258 = Multiply(x=w457, y=w453) -> (x*y=w470:fxp<+/-,34,9>)
    "Sin omega_p" <- w470
    n259 = Negate(x=w467) -> (-x=w466:fxp<+/-,35,19>)
    n260 = Multiply(x=w470, y=w454) -> (x*y=w469:fxp<+/-,33,15>)
    n261 = Multiply(x=w466, y=w456) -> (x*y=w465:fxp<+/-,35,19>)
    n262 = Multiply(x=w463, y=w469) -> (x*y=→"Dpr_sin_d":fxp<+/-,33,15>)
    n263 = Multiply(x=w458, y=w465) -> (x*y=→"Dpr_sin_dd":fxp<+/-,35,20>)
    n264 = Multiply(x="Sin magnitude_p", y=w458) -> (x*y=w461:fxp<+/-,37,8>)
    n265 = Add(x=w461, y="Sin offset_p") -> (x+y=→"Dpr_sin":fxp<+/-,37,8>)
  }
  n266 = while "Time reset" {
    shift-right: [w568] -> _
    shift-left: _ -> [w569]
    shift-right: [w563] -> _
    shift-left: _ -> [w564]
    stop <- FALSE stop-if-true
    n267 = local read "Stop motor_y"() -> (w570:bool)
    n268 = call "Tick Count3"() -> ("Tick Count(uSec)"=w568:u32)
    n269 = Subtract(x=w568, y=w569) -> (x-y=w567:u32)
    n270 = Add(x=w564, y=w567) -> (x+y=w566:u32)
    n271 = Select(t=u32 0, s=w570, f=w566) -> (s? t:f=w563:u32)
    n272 = To Fixed-Point(number=w563) -> (fixed-point=w562:fxp<+,32,32>)  [unwired: 1 in]
    n273 = Multiply(x=fxp<+,20,-18> 1.0000003385357559e-06, y=w562) -> (x*y=→"Time now(s)":fxp<+,52,14>)
  }
  n274 = while "Ini" {
    stop <- FALSE stop-if-true
    n275 = case shown="True" "Ini coe." {
      frame False {
      }
      frame True {
        w578 = T2 20 items=["50.000 kS/s (NI 9237)"=1, "25.000 kS/s (NI 9237)"=2, "16.667 kS/s (NI 9237)"=3, "12.500 kS/s (NI 9237)"=4, "10.000 kS/s (NI 9237)"=5, "8.333 kS/s (NI 9237)"=6, "7.143 kS/s (NI 9237)"=7, "6.250 kS/s (NI 9237)"=8, "5.556 kS/s (NI 9237)"=9, "5.000 kS/s (NI 9237)"=10, "4.545 kS/s (NI 9237)"=11, "4.167 kS/s (NI 9237)"=12, "3.846 kS/s (NI 9237)"=13, "3.571 kS/s (NI 9237)"=14, "3.333 kS/s (NI 9237)"=15, "3.125 kS/s (NI 9237)"=16, "2.941 kS/s (NI 9237)"=17, "2.778 kS/s (NI 9237)"=18, "2.632 kS/s (NI 9237)"=19, "2.500 kS/s (NI 9237)"=20, "2.381 kS/s (NI 9237)"=21, "2.273 kS/s (NI 9237)"=22, "2.174 kS/s (NI 9237)"=23, "2.083 kS/s (NI 9237)"=24, "2.000 kS/s (NI 9237)"=25, "1.923 kS/s (NI 9237)"=26, "1.852 kS/s (NI 9237)"=27, "1.786 kS/s (NI 9237)"=28, "1.724 kS/s (NI 9237)"=29, "1.667 kS/s (NI 9237)"=30, "1.613 kS/s (NI 9237)"=31] ("Data Rate")
        w595 = i16 0 items=["Step", "Sine"] ("Command_p")
        w596 = i16 2 items=["Raw", "Avg.", "Avg. w. filter"] ("Strain selection_p")
        w597 = i16 0 items=["Step", "Sine"] ("Command_y")
        w598 = i16 2 items=["Raw", "Avg.", "Avg. w. filter"] ("Strain selection_y")
        w600 = fxp<+/-,25,-10> 5.851034075021744e-07  # S/F coeff_p
        w599 = fxp<+/-,25,-10> 1.0477961041033268e-06  # S/F coeff_y
        w606 = i16 0 items=["Backward", "Forward"] ("Drive mode")
        n276 = local write "Sin wave freq._y (Hz)"(fxp<+/-,32,6> 1.0 ("Sin wave freq. (Hz)")) -> ()
        n277 = local write "Sin magnitude_y"(fxp<+/-,22,7> 5.0 ("Sin magnitude")) -> ()
        n278 = local write "fy_tolorance"(fxp<+,22,6> 5.0 ("f_tolorance")) -> ()
        n279 = local write "Sin offset_y"(fxp<+/-,38,9> 0.0 ("Sin offset")) -> ()
        n280 = local write "Dyr_step"(fxp<+/-,22,7> 0.0 ("Dr")) -> ()
        n281 = local write "Kp_y"(fxp<+/-,36,9> 30.0 ("Kp")) -> ()
        n282 = local write "Kd_y"(fxp<+/-,36,9> 0.0 ("Kd")) -> ()
        n283 = local write "Kv_y"(fxp<+/-,22,8> 0.0 ("Kv")) -> ()
        n284 = local write "Bv_y"(fxp<+/-,22,8> 0.0 ("Bv")) -> ()
        n285 = local write "Ki_y"(fxp<+/-,36,9> 0.0 ("Ki")) -> ()
        n286 = local write "S/F coeff_p"(w600) -> ()
        n287 = local write "S/F coeff_y"(w599) -> ()
        n288 = local write "Data Rate"(w578) -> ()
        n289 = local write "dFy_add"(FALSE ("dF_add")) -> ()
        n290 = local write "dFp_add"(FALSE ("dFp_add")) -> ()
        n291 = local write "Sin wave freq._p (Hz)"(fxp<+/-,32,6> 1.0 ("Sin wave freq._p (Hz)")) -> ()
        n292 = local write "Sin magnitude_p"(fxp<+/-,21,6> 5.0 ("Sin magnitude_p")) -> ()
        n293 = local write "fp_tolorance"(fxp<+,22,6> 5.0 ("fp_tolorance")) -> ()
        n294 = local write "Sin offset_p"(fxp<+/-,22,7> 0.0 ("Sin offset_p")) -> ()
        n295 = local write "Dpr_step"(fxp<+/-,22,7> 0.0 ("Dpr_step")) -> ()
        n296 = local write "Kp_p"(fxp<+/-,36,9> 30.0 ("Kp_p")) -> ()
        n297 = local write "Kd_p"(fxp<+/-,36,9> 0.0 ("Kd_p")) -> ()
        n298 = local write "Kv_p"(fxp<+/-,22,8> 0.0 ("Kv_p")) -> ()
        n299 = local write "Bv_p"(fxp<+/-,22,8> 0.0 ("Bv_p")) -> ()
        n300 = local write "Ki_p"(fxp<+/-,36,9> 0.0 ("Ki_p")) -> ()
        n301 = local write "Strain selection_p"(w596) -> ()
        n302 = local write "Strain selection_y"(w598) -> ()
        n303 = local write "Command_p"(w595) -> ()
        n304 = local write "Command_y"(w597) -> ()
        n305 = local write "Drive mode"(w606) -> ()
        n306 = local write "Dp_d_M_avg_Tc (uSec)"(u32 1000 ("D_d_M_avg_Tc (uSec)")) -> ()
        n307 = local write "Dy_d_M_avg_Tc (uSec)"(1000 ("Dy_d_M_avg_Tc (uSec)")) -> ()
        n308 = local write "Belt_out_p"(fxp<+/-,7,7> 36.0 ("Belt_op")) -> ()
        n309 = local write "Belt_out_y"(fxp<+/-,7,7> 22.0 ("Belt_oy")) -> ()
        n310 = local write "Belt_in_p"(fxp<+/-,6,6> 14.0 ("Belt_mp")) -> ()
        n311 = local write "Belt_in_y"(fxp<+/-,6,6> 16.0 ("Belt_my")) -> ()
        n312 = local write "mt0_p1"(u32 40000000 ("mt0_p1")) -> ()
        n313 = local write "mt0_p2"(u32 40000000 ("mt0_p2")) -> ()
        n314 = local write "mt0_y1"(u32 40000000 ("mt0_y1")) -> ()
        n315 = local write "mt0_y2"(u32 40000000 ("mt0_y2")) -> ()
      }
    }
  }
  n316 = while "FIFO" {
    stop <- FALSE stop-if-true
    n317 = flat-sequence {
      frame #0 {
        n318 = call "Loop Timer"("Count(uSec)"=u32 1000) -> ()  [unwired: 1 out]
      }
      frame #1 {
        n319 = case shown="2" "FIFO" {
          tunnel: [w649 w665 w681] -> w633
          tunnel: [w648 w664 w680] -> w632
          tunnel: [w647 w663 w679] -> w631
          tunnel: [w646 w662 w678] -> w630
          tunnel: [w643 w661 w675] -> w628
          tunnel: [w644 w660 w676] -> w627
          tunnel: [w645 w659 w677] -> w626
          tunnel: [w641 w658 w673] -> w625
          tunnel: [w640 w657 w672] -> w624
          tunnel: [w639 w656 w671] -> w623
          tunnel: [w638 w655 w670] -> w622
          tunnel: [w637 w654 w669] -> w621
          tunnel: [w636 w653 w668] -> w620
          tunnel: [w635 w652 w667] -> w619
          tunnel: [w634 fxp<+,1,1> 0.0 ("element") w666] -> w618
          tunnel: [w642 fxp<+,1,1> 0.0 w674] -> w616
          frame 0 {
            # "Pitch"
            n320 = local read "omega_p (Mavg w. f)"() -> (w635:fxp<+/-,36,14>)
            n321 = local read "omega_p1 (Mavg)"() -> (w643:fxp<+/-,36,14>)
            n322 = local read "Dp1_d (Mavg)"() -> (w634:fxp<+/-,36,14>)
            n323 = local read "Encoder Position_p1"() -> (w649:i32)
            n324 = local read "Encoder Position_p2"() -> (w648:i32)
            n325 = local read "D_p1"() -> (w647:fxp<+/-,32,7>)
            n326 = local read "D_p2"() -> (w646:fxp<+/-,32,7>)
            n327 = local read "omega_p1 (T)"() -> (w645:fxp<+/-,36,13>)
            n328 = local read "omega_p2 (T)"() -> (w644:fxp<+/-,36,13>)
            n329 = local read "rad_p1"() -> (w642:fxp<+/-,33,20>)
            n330 = local read "rad_p2"() -> (w641:fxp<+/-,33,20>)
            n331 = local read "Force_p"() -> (w640:fxp<+/-,32,10>)
            n332 = local read "Raw Strain_p"() -> (w639:fxp<+/-,36,4>)
            n333 = local read "Strain_p (Avg8)"() -> (w638:fxp<+/-,36,4>)
            n334 = local read "Strain_p (Avg8 w. f)"() -> (w637:fxp<+/-,36,8>)
            n335 = local read "Dp_d (mm/s)"() -> (w636:fxp<+/-,36,13>)
          }
          frame 1, Default {
            # "imp ctrl"
            n336 = local read "D_y(mm)"() -> (w665:fxp<+/-,32,7>)
            n337 = local read "Raw Strain_y"() -> (w664:fxp<+/-,36,4>)
            n338 = local read "Strain_y (Avg8)"() -> (w663:fxp<+/-,36,4>)
            n339 = local read "Strain_y (Avg8 w. f)"() -> (w662:fxp<+/-,36,8>)
            n340 = local read "Force_y"() -> (w659:fxp<+/-,32,10>)
            n341 = local read "Dy_d (T)"() -> (w660:fxp<+/-,36,13>)
            n342 = local read "Fy_dc"() -> (w661:fxp<+/-,32,10>)
            n343 = local read "D_p(mm)"() -> (w658:fxp<+/-,32,7>)
            n344 = local read "Raw Strain_p"() -> (w657:fxp<+/-,36,4>)
            n345 = local read "Strain_p (Avg8)"() -> (w656:fxp<+/-,36,4>)
            n346 = local read "Strain_p (Avg8 w. f)"() -> (w655:fxp<+/-,36,8>)
            n347 = local read "Force_p"() -> (w654:fxp<+/-,32,10>)
            n348 = local read "Dp_d (mm/s)"() -> (w653:fxp<+/-,36,13>)
            n349 = local read "Fp_dc"() -> (w652:fxp<+/-,32,10>)
          }
          frame 2 {
            # "Yaw"
            n350 = local read "omega_y (Mavg w. f.)"() -> (w667:fxp<+/-,36,14>)
            n351 = local read "omega_y1 (Mavg)"() -> (w675:fxp<+/-,36,14>)
            n352 = local read "Dy1_d (Mavg)"() -> (w666:fxp<+/-,36,14>)
            n353 = local read "Encoder Position_y1"() -> (w681:i32)
            n354 = local read "Encoder Position_y2"() -> (w680:i32)
            n355 = local read "D_y1"() -> (w679:fxp<+/-,32,7>)
            n356 = local read "D_y2"() -> (w678:fxp<+/-,32,7>)
            n357 = local read "omega_y1 (T)"() -> (w677:fxp<+/-,36,13>)
            n358 = local read "omega_y2 (T)"() -> (w676:fxp<+/-,36,13>)
            n359 = local read "rad_y1"() -> (w674:fxp<+/-,33,20>)
            n360 = local read "rad_y2"() -> (w673:fxp<+/-,33,20>)
            n361 = local read "Force_y"() -> (w672:fxp<+/-,32,10>)
            n362 = local read "Raw Strain_y"() -> (w671:fxp<+/-,36,4>)
            n363 = local read "Strain_y (Avg8)"() -> (w670:fxp<+/-,36,4>)
            n364 = local read "Strain_y (Avg8 w. f)"() -> (w669:fxp<+/-,36,8>)
            n365 = local read "Dy_d (mm/s)"() -> (w668:fxp<+/-,36,13>)
          }
        }
        n366 = Build Array(w633, w632, w631, w630, w626, w627, w628, w616, w625, w624, w623, w622, w621, w620, w619, w618) -> (w617:fxp<+/-,64,32>[])
        n367 = xnode ("FIFO Write")("Element"=w617, "Timeout"=0) -> ()  [unwired: 1 in, 2 out]
      }
    }
  }
  n368 = while "PID force controller_y" {
    stop <- FALSE stop-if-true
    n369 = local read "Force_y"() -> (w683:fxp<+/-,32,10>)
    n370 = local read "fyt_d"() -> (w692:fxp<+/-,36,18>)
    n371 = local read "Fr_y"() -> (w684:fxp<+/-,32,10>)
    n372 = Subtract(x=w684, y=w683) -> (x-y=w682:fxp<+/-,33,11>)
    "fy_tilde" <- w682
    n373 = Absolute Value(x=w682) -> (abs(x)=w699:fxp<+,32,10>)
    n374 = local read "fyt_i"() -> (w688:fxp<+/-,36,16>)
    n375 = Multiply(x="Kp_y", y=w682) -> (x*y=w690:fxp<+/-,64,23>)
    n376 = Multiply(x="Kd_y", y=w692) -> (x*y=w691:fxp<+/-,64,27>)
    n377 = Multiply(x="Ki_y", y=w688) -> (x*y=w686:fxp<+/-,64,25>)
    n378 = Add(x=w690, y=w691) -> (x+y=w687:fxp<+/-,64,28>)
    n379 = Greater?(x=w699, y="fy_tolorance") -> (0:w697:bool)
    n380 = Add(x=w687, y=w686) -> (x+y=w685:fxp<+/-,36,16>)
    n381 = Select(t=w685, s=w697, f=fxp<+/-,51,14> 0.0) -> (s? t:f=→"Fy_PID":fxp<+/-,53,16>)
  }
  n382 = for {
    N: w2 -> [_]
    tunnel: [w702] -> w4 mode=indexing
    tunnel: [w701] -> w3 mode=indexing
    tunnel: [w701] -> w1
    n383 = local read "Dy_d_M_avg_Tc (uSec)"() -> (w701:i32)
    n384 = local read "Encoder Position_p2"() -> (w702:i32)
    n385 = call "Wait5"("Count(uSec)"=w701) -> ()  [unwired: 1 out]
  }
  n386 = while {
    tunnel: w24 -> [w747]
    tunnel: [w721] -> w17
    shift-right: [w745] -> _
    shift-left: _ -> [w746]
    shift-right: [w741] -> _
    shift-left: _ -> [w742]
    shift-right: [w736] -> _
    shift-left: _ -> [w735]
    shift-right: [w735] -> _
    shift-left: _ -> [w734]
    shift-right: [w734] -> _
    shift-left: _ -> [w733]
    shift-right: [w733] -> _
    shift-left: _ -> [w732]
    shift-right: [w732] -> _
    shift-left: _ -> [w731]
    shift-right: [w731] -> _
    shift-left: _ -> [w730]
    shift-right: [w730] -> _
    shift-left: _ -> [w729]
    tunnel: w24 -> [w725]
    shift-right: [w718] -> _
    shift-left: _ -> [w719]
    shift-right: [w714] -> _
    shift-left: _ -> [w713]
    shift-right: [w713] -> _
    shift-left: _ -> [w712]
    shift-right: [w712] -> _
    shift-left: _ -> [w711]
    shift-right: [w711] -> _
    shift-left: _ -> [w710]
    shift-right: [w710] -> _
    shift-left: _ -> [w709]
    shift-right: [w709] -> _
    shift-left: _ -> [w708]
    shift-right: [w708] -> _
    shift-left: _ -> [w707]
    stop <- w722 stop-if-true
    w716 = fxp<+,20,2> 2.115001678466797  # Gage Factor
    n387 = xnode "FPGA I/O Node"("error in"=w747) -> ("error out"=w721:errorcluster, "Mod6/AI2"=w743:fxp<+/-,24,-4>)  [unwired: 1 in, 1 out]
    n388 = xnode "FPGA I/O Node"("error in"=w725) -> ("error out"=w723:errorcluster, "Mod6/AI3"=w717:fxp<+/-,24,-4>)  [unwired: 1 in, 1 out]
    n389 = Or(x=w721, y="Stop (Strain)") -> (x .or. y?=w724:bool)
    n390 = Select(t=w717, s="Strain gage reset_p", f=w719) -> (s? t:f=w718:fxp<+/-,24,-4>)
    n391 = Select(t=w743, s="Strain gage reset_y", f=w746) -> (s? t:f=w745:fxp<+/-,24,-4>)
    n392 = Or(x=w724, y=w723) -> (x .or. y?=w722:bool)
    n393 = Subtract(x=w717, y=w718) -> (x-y=w715:fxp<+/-,30,-3>)
    "Mod6/AI3" <- w715
    n394 = Subtract(x=w743, y=w745) -> (x-y=w744:fxp<+/-,30,-3>)
    "Mod6/AI2" <- w744
    n395 = Multiply(x=w716, y=w744) -> (x*y=w736:fxp<+/-,41,6>)
    "Raw Strain_y" <- w736
    n396 = Multiply(x=w716, y=w715) -> (x*y=w714:fxp<+/-,50,-1>)
    "Raw Strain_p" <- w714
    n397 = call "average_v2.vi"("Numeric 8"=w707, "Numeric"=w714, "Numeric 7"=w708, "Numeric 2"=w713, "Numeric 6"=w709, "Numeric 5"=w710, "Numeric 4"=w711, "Numeric 3"=w712) -> ("Mean (8pt)"=w706:fxp<+/-,32,4>)  [unwired: 1 in, 2 out]
    "Strain_p (Avg8)" <- w706
    n398 = call "average_v2.vi"("Numeric 8"=w729, "Numeric"=w736, "Numeric 7"=w730, "Numeric 2"=w735, "Numeric 6"=w731, "Numeric 5"=w732, "Numeric 4"=w733, "Numeric 3"=w734) -> ("Mean (8pt)"=w728:fxp<+/-,32,4>)  [unwired: 1 in, 2 out]
    "Strain_y (Avg8)" <- w728
    n399 = call "Tick Count"() -> ("Tick Count(uSec)"=w741:u32)
    n400 = xnode "Butterworth Filter"("input data"=w706, "scaled coefficients"="Strain_p Avg.8 coeff.") -> ("output data"=→"Strain_p (Avg8 w. f)":fxp<+/-,36,8>)  [unwired: 1 in]
    n401 = xnode "Butterworth Filter"("input data"=w728, "scaled coefficients"="Strain_y Avg8 coeff.") -> ("output data"=→"Strain_y (Avg8 w. f)":fxp<+/-,32,4>)  [unwired: 1 in]
    n402 = Subtract(x=w741, y=w742) -> (x-y=w739:fxp<+/-,32,16>)
    n403 = Divide(x=fxp<+,7,10> 1000.0, y=w739) -> (x/y=→"Loop rate (kHz)":fxp<+/-,40,27>)
  }
  n404 = for {
    N: w5 -> [_]
    tunnel: [w766] -> w8 mode=indexing
    tunnel: [w765] -> w7 mode=indexing
    tunnel: [w764] -> w6
    n405 = local read "Dy_d_M_avg_Tc (uSec)"() -> (w764:i32)
    n406 = local read "Encoder Position_y2"() -> (w766:i32)
    n407 = call "Wait4"("Count(uSec)"=w764) -> ("Tick Count(uSec)"=w765:u32)
  }
  n408 = for {
    N: w13 -> [_]
    tunnel: [w769] -> w12 mode=indexing
    tunnel: [w768] -> w11 mode=indexing
    tunnel: ["Dy_d_M_avg_Tc (uSec)"] -> w10
    n409 = local read "Encoder Position_y1"() -> (w768:i32)
    n410 = call "Wait3"("Count(uSec)"="Dy_d_M_avg_Tc (uSec)") -> ("Tick Count(uSec)"=w769:u32)
  }
  n411 = for {
    N: w16 -> [_]
    tunnel: ["Dp_d_M_avg_Tc (uSec)"] -> w9
    tunnel: [w771] -> w15 mode=indexing
    tunnel: [w770] -> w14 mode=indexing
    n412 = local read "Encoder Position_p1"() -> (w770:i32)
    n413 = call "Wait2"("Count(uSec)"="Dp_d_M_avg_Tc (uSec)") -> ("Tick Count(uSec)"=w771:u32)
  }
  n414 = while "Omega_p2 (Mavg)" {
    shift-right: _ -> [_]
    shift-left: w4 -> [w796]
    shift-right: _ -> [_]
    shift-left: w3 -> [w794]
    shift-right: [w777] -> _
    shift-left: _ -> [w773]
    tunnel: w2 -> [w792]
    tunnel: w1 -> [w797]
    stop <- FALSE stop-if-true
    w778 = fxp<+/-,27,3> 3.1415926814079285  # pi
    w784 = fxp<+,32,0> 0.1953125  # 800/4096
    w789 = fxp<+/-,32,0> 0.3183098859153688  # L/2/pi
    n415 = call "Tick Count9"() -> ("Tick Count(uSec)"=w791:u32)
    n416 = Index Array(array=w794, index=0) -> (element=w793:i32)
    n417 = Index Array(array=w796, index=0) -> (element=w795:i32)
    n418 = Multiply(x=w792, y=w797) -> (x*y=w800:i32)
    n419 = Add(x=w800, y=w793) -> (x+y=w799:i32)
    n420 = Greater Or Equal?(x=w791, y=w799) -> (x >= y?=w798:bool)
    n421 = case shown="True" w798 {
      tunnel: w796 -> [w804 w818]
      tunnel: w795 -> [_ w810]
      tunnel: w794 -> [w805 w819]
      tunnel: w793 -> [_ w820]
      tunnel: w792 -> [_ w817]
      tunnel: w791 -> [_ w821]
      tunnel: [w804 w808] -> _
      tunnel: [w805 w807] -> _
      tunnel: [w803 w806] -> w777
      tunnel: w773 -> [w803 _]
      frame False {
      }
      frame True {
        n422 = local read "Encoder Position_p2"() -> (w809:i32)
        n423 = Subtract(x=w821, y=w820) -> (x-y=w822:u32)
        n424 = Insert Into Array(array=w819) -> (w824:i32[])  [unwired: 2 in]
        n425 = Subtract(x=w809, y=w810) -> (x-y=w814:i32)
        n426 = Insert Into Array(array=w818, index=w817, new element=w809) -> (w825:i32[])
        n427 = To Fixed-Point(number=w822) -> (fixed-point=w811:fxp<+,32,32>)  [unwired: 1 in]
        n428 = Multiply(x=w814, y=2500) -> (x*y=w815:i32)
        n429 = To Fixed-Point(number=w815) -> (fixed-point=w816:fxp<+/-,32,32>)  [unwired: 1 in]
        n430 = Delete From Array(array=w824, length=1, index=0) -> (array with subset deleted=w807:i32[])  [unwired: 1 out]
        n431 = Delete From Array(array=w825, length=1, index=0) -> (array with subset deleted=w808:i32[])  [unwired: 1 out]
        n432 = Divide(x=w816, y=w811) -> (x/y=w806:fxp<+/-,56,22>)
      }
    }
    n433 = local read "Mag. factor_p"() -> (w783:fxp<+/-,20,3>)
    n434 = local read "Mag. encoder_y"() -> (w781:bool)
    n435 = local read "Belt_in_p"() -> (w786:fxp<+/-,6,6>)
    n436 = local read "Belt_out_p"() -> (w785:fxp<+/-,7,7>)
    n437 = Divide(x=w784, y=w783) -> (x/y=w782:fxp<+/-,32,1>)
    n438 = Multiply(x=w778, y=w777) -> (x*y=w780:fxp<+/-,64,25>)
    n439 = Select(t=w782, s=w781, f=fxp<+/-,2,2> 1.0) -> (s? t:f=w776:fxp<+/-,33,2>)
    n440 = Multiply(x=w789, y=w786) -> (x*y=w790:fxp<+/-,38,6>)
    n441 = Multiply(x=w776, y=w780) -> (x*y=→"omega_p2 (Mavg)":fxp<+/-,64,27>)
    n442 = Divide(x=w790, y=w785) -> (x/y=w788:fxp<+/-,45,6>)
    n443 = Multiply(x=w788) -> (x*y=→"Dp2_d (Mavg)":fxp<+/-,64,10>)  [unwired: 1 in]
  }
  n444 = while "Omega_y1 (Mavg)" {
    tunnel: w13 -> [w851]
    shift-right: [w849] -> _
    shift-left: w12 -> [w854]
    shift-right: [w848] -> _
    shift-left: w11 -> [w850]
    shift-right: [w843] -> _
    shift-left: _ -> [w847]
    tunnel: w10 -> [w842]
    stop <- FALSE stop-if-true
    w830 = fxp<+/-,32,0> 0.3183098859153688  # L/2/pi
    w839 = fxp<+,32,0> 0.1953125  # 800/4096
    w845 = fxp<+/-,27,3> 0.007853984832763672  # 2*pi/800
    n445 = call "Tick Count6"() -> ("Tick Count(uSec)"=w855:u32)
    n446 = Index Array(array=w854, index=0) -> (element=w853:u32)
    n447 = Index Array(array=w850, index=0) -> (element=w852:i32)
    n448 = Multiply(x=w851, y=w842) -> (x*y=w857:i32)
    n449 = Add(x=w857, y=w853) -> (x+y=w856:u32)
    n450 = Greater Or Equal?(x=w855, y=w856) -> (x >= y?=w846:bool)
    n451 = case shown="True" w846 {
      tunnel: w855 -> [_ w878]
      tunnel: w851 -> [_ w875]
      tunnel: w854 -> [w862 w877]
      tunnel: w853 -> [_ w876]
      tunnel: w852 -> [_ w872]
      tunnel: w850 -> [w861 w874]
      tunnel: [w860 w870] -> w843
      tunnel: [w862 w869] -> w849
      tunnel: [w861 w868] -> w848
      tunnel: w847 -> [w860 _]
      frame False {
      }
      frame True {
        # "count/s"
        n452 = local read "Encoder Position_y1"() -> (w871:i32)
        n453 = Subtract(x=w878, y=w876) -> (x-y=w879:u32)
        n454 = Insert Into Array(array=w877, new element=w878) -> (w881:u32[])  [unwired: 1 in]
        n455 = Subtract(x=w871, y=w872) -> (x-y=w866:i32)
        n456 = Insert Into Array(array=w874, index=w875, new element=w871) -> (w882:i32[])
        n457 = To Fixed-Point(number=w879) -> (fixed-point=w865:fxp<+,32,32>)  [unwired: 1 in]
        n458 = To Fixed-Point(number=w866) -> (fixed-point=w873:fxp<+/-,32,32>)  [unwired: 1 in]
        n459 = Divide(x=w865, y=fxp<+,32,32> 1000000.0) -> (x/y=w864:fxp<+/-,64,32>)
        n460 = Delete From Array(array=w881, length=1, index=0) -> (array with subset deleted=w869:u32[])  [unwired: 1 out]
        n461 = Delete From Array(array=w882, length=1, index=0) -> (array with subset deleted=w868:i32[])  [unwired: 1 out]
        n462 = Divide(x=w873, y=w864) -> (x/y=w870:fxp<+/-,56,22>)
      }
    }
    n463 = local read "Mag. factor_y"() -> (w838:fxp<+/-,20,3>)
    n464 = local read "Mag. encoder_y"() -> (w841:bool)
    n465 = local read "Belt_in_y"() -> (w832:fxp<+/-,6,6>)
    n466 = Multiply(x=w845, y=w843) -> (x*y=w835:fxp<+/-,64,25>)
    n467 = Divide(x=w839, y=w838) -> (x/y=w837:fxp<+/-,32,1>)
    n468 = local read "Belt_out_y"() -> (w833:fxp<+/-,7,7>)
    n469 = Select(t=w837, s=w841, f=fxp<+/-,2,2> 1.0) -> (s? t:f=w836:fxp<+/-,33,2>)
    n470 = Multiply(x=w830, y=w832) -> (x*y=w831:fxp<+/-,38,6>)
    n471 = Multiply(x=w836, y=w835) -> (x*y=w834:fxp<+/-,64,27>)
    "omega_y1 (Mavg)" <- w834
    n472 = Divide(x=w831, y=w833) -> (x/y=w829:fxp<+/-,45,6>)
    n473 = Multiply(x=w829, y=w834) -> (x*y=→"Dy1_d (Mavg)":fxp<+/-,64,32>)
  }
  n474 = while "Omega_p1 (Mavg)" {
    tunnel: w16 -> [w908]
    shift-right: [w906] -> _
    shift-left: w15 -> [w911]
    shift-right: [w905] -> _
    shift-left: w14 -> [w907]
    shift-right: [w904] -> _
    shift-left: _ -> [w903]
    tunnel: w9 -> [w901]
    stop <- FALSE stop-if-true
    w890 = fxp<+/-,27,3> 3.1415926814079285  # pi
    w892 = fxp<+,32,0> 0.1953125  # 800/4096
    w889 = fxp<+/-,32,0> 0.3183098859153688  # L/2/pi
    n475 = call "Tick Count5"() -> ("Tick Count(uSec)"=w912:u32)
    n476 = Index Array(array=w911, index=0) -> (element=w910:u32)
    n477 = Index Array(array=w907, index=0) -> (element=w909:i32)
    n478 = Multiply(x=w908, y=w901) -> (x*y=w914:i32)
    n479 = Add(x=w914, y=w910) -> (x+y=w913:u32)
    n480 = Greater Or Equal?(x=w912, y=w913) -> (x >= y?=w902:bool)
    n481 = case shown="True" w902 {
      tunnel: w912 -> [_ w935]
      tunnel: w908 -> [_ w932]
      tunnel: w911 -> [w919 w934]
      tunnel: w910 -> [_ w933]
      tunnel: w909 -> [_ w929]
      tunnel: w907 -> [w918 w931]
      tunnel: [w917 w927] -> w904
      tunnel: [w919 w926] -> w906
      tunnel: [w918 w925] -> w905
      tunnel: w903 -> [w917 _]
      frame False {
      }
      frame True {
        n482 = local read "Encoder Position_p1"() -> (w928:i32)
        n483 = Subtract(x=w935, y=w933) -> (x-y=w936:u32)
        n484 = Subtract(x=w928, y=w929) -> (x-y=w921:i32)
        n485 = Insert Into Array(array=w934, new element=w935) -> (w938:u32[])  [unwired: 1 in]
        n486 = Insert Into Array(array=w931, index=w932, new element=w928) -> (w939:i32[])
        n487 = To Fixed-Point(number=w936) -> (fixed-point=w923:fxp<+,32,32>)  [unwired: 1 in]
        n488 = Multiply(x=w921, y=2500) -> (x*y=w922:i32)
        n489 = To Fixed-Point(number=w922) -> (fixed-point=w930:fxp<+/-,32,32>)  [unwired: 1 in]
        n490 = Delete From Array(array=w938, length=1, index=0) -> (array with subset deleted=w926:u32[])  [unwired: 1 out]
        n491 = Delete From Array(array=w939, length=1, index=0) -> (array with subset deleted=w925:i32[])  [unwired: 1 out]
        n492 = Divide(x=w930, y=w923) -> (x/y=w927:fxp<+/-,56,22>)
      }
    }
    n493 = local read "Mag. factor_p"() -> (w893:fxp<+/-,20,3>)
    n494 = local read "Mag. encoder_p"() -> (w900:bool)
    n495 = local read "Belt_in_p"() -> (w897:fxp<+/-,6,6>)
    n496 = Divide(x=w892, y=w893) -> (x/y=w891:fxp<+/-,32,1>)
    n497 = local read "Belt_out_p"() -> (w896:fxp<+/-,7,7>)
    n498 = Multiply(x=w890, y=w904) -> (x*y=w898:fxp<+/-,64,25>)
    n499 = Select(t=w891, s=w900, f=fxp<+/-,2,2> 1.0) -> (s? t:f=w885:fxp<+/-,33,2>)
    n500 = Multiply(x=w889, y=w897) -> (x*y=w895:fxp<+/-,38,6>)
    n501 = Multiply(x=w885, y=w898) -> (x*y=w888:fxp<+/-,64,27>)
    "omega_p1 (Mavg)" <- w888
    n502 = Divide(x=w895, y=w896) -> (x/y=w887:fxp<+/-,45,6>)
    n503 = Multiply(x=w887, y=w888) -> (x*y=→"Dp1_d (Mavg)":fxp<+/-,64,32>)
  }
  n504 = while "Omega_y2 (Mavg)" {
    shift-right: _ -> [_]
    shift-left: w7 -> [w965]
    shift-right: _ -> [_]
    shift-left: w8 -> [w967]
    tunnel: w6 -> [w963]
    tunnel: w5 -> [w961]
    shift-right: [w945] -> _
    shift-left: _ -> [w959]
    stop <- FALSE stop-if-true
    w948 = fxp<+/-,27,3> 0.007853984832763672  # 2*pi/800
    w952 = fxp<+,32,0> 0.1953125  # 800/4096
    w957 = fxp<+/-,32,0> 0.3183098859153688  # L/2/pi
    n505 = call "Tick Count8"() -> ("Tick Count(uSec)"=w966:u32)
    n506 = Index Array(array=w965, index=0) -> (element=w964:u32)
    n507 = Index Array(array=w967, index=0) -> (element=w962:i32)
    n508 = Multiply(x=w961, y=w963) -> (x*y=w969:i32)
    n509 = Add(x=w969, y=w964) -> (x+y=w968:u32)
    n510 = Greater Or Equal?(x=w966, y=w968) -> (x >= y?=w960:bool)
    n511 = case shown="True" w960 {
      tunnel: w967 -> [w972 w985]
      tunnel: w966 -> [_ w988]
      tunnel: w965 -> [w973 w987]
      tunnel: w964 -> [_ w986]
      tunnel: w962 -> [_ w975]
      tunnel: w961 -> [_ w984]
      tunnel: [w973 w983] -> _
      tunnel: [w972 w982] -> _
      tunnel: [w974 w977] -> w945
      tunnel: w959 -> [w974 _]
      frame False {
      }
      frame True {
        n512 = local read "Encoder Position_y2"() -> (w976:i32)
        n513 = Subtract(x=w988, y=w986) -> (x-y=w991:u32)
        n514 = Insert Into Array(array=w987, new element=w988) -> (w993:u32[])  [unwired: 1 in]
        n515 = Insert Into Array(array=w985, index=w984, new element=w976) -> (w994:i32[])
        n516 = Subtract(x=w976, y=w975) -> (x-y=w980:i32)
        n517 = To Fixed-Point(number=w991) -> (fixed-point=w990:fxp<+,32,32>)  [unwired: 1 in]
        n518 = To Fixed-Point(number=w980) -> (fixed-point=w981:fxp<+/-,32,32>)  [unwired: 1 in]
        n519 = Divide(x=w990, y=fxp<+,32,32> 1000000.0) -> (x/y=w979:fxp<+/-,64,32>)
        n520 = Delete From Array(array=w993, length=1, index=0) -> (array with subset deleted=w983:u32[])  [unwired: 1 out]
        n521 = Delete From Array(array=w994, length=1, index=0) -> (array with subset deleted=w982:i32[])  [unwired: 1 out]
        n522 = Divide(x=w981, y=w979) -> (x/y=w977:fxp<+/-,56,22>)
      }
    }
    n523 = local read "Mag. factor_y"() -> (w951:fxp<+/-,20,3>)
    n524 = local read "Mag. encoder_y"() -> (w949:bool)
    n525 = local read "Belt_in_y"() -> (w954:fxp<+/-,6,6>)
    n526 = Divide(x=w952, y=w951) -> (x/y=w950:fxp<+/-,32,1>)
    n527 = local read "Belt_out_y"() -> (w953:fxp<+/-,7,7>)
    n528 = Multiply(x=w948, y=w945) -> (x*y=w947:fxp<+/-,64,25>)
    n529 = Select(t=w950, s=w949, f=fxp<+/-,2,2> 1.0) -> (s? t:f=w944:fxp<+/-,33,2>)
    n530 = Multiply(x=w957, y=w954) -> (x*y=w958:fxp<+/-,38,6>)
    n531 = Multiply(x=w944, y=w947) -> (x*y=→"omega_y2 (Mavg)":fxp<+/-,64,27>)
    n532 = Divide(x=w958, y=w953) -> (x/y=w956:fxp<+/-,45,6>)
    n533 = Multiply(x=w956) -> (x*y=→"Dy2_d (Mavg)":fxp<+/-,64,10>)  [unwired: 1 in]
  }
  n534 = while "Quadrature drive_p" {
    stop <- FALSE stop-if-true
    n535 = local read "dFp_PID"() -> (w998:fxp<+/-,36,18>)
    n536 = local read "omega_p (rad/s)"() -> (w1004:fxp<+/-,36,13>)
    n537 = local read "Fp_PID"() -> (w999:fxp<+/-,36,16>)
    n538 = Select(t=w998, s="dFp_add", f=fxp<+,1,1> 0.0) -> (s? t:f=w1002:fxp<+/-,36,18>)
    n539 = call "Oriental_step_motor_PKP225.vi"("F_Threshold"=fxp<+,12,12> 10.0, "dFmr"=w1002, "omega"=w1004, "Fmr"=w999) -> ("vq_F"=→"vq_p_F":fxp<+/-,20,5>, "vd_F"=→"vd_p_F":fxp<+/-,20,5>)  [unwired: 6 in]
  }
  n540 = while "PID force controller_p" {
    shift-right: [w1011] -> _
    shift-left: _ -> [w1010]
    stop <- FALSE stop-if-true
    n541 = local read "Force_p"() -> (w1023:fxp<+/-,32,10>)
    n542 = local read "fpt_d"() -> (w1019:fxp<+/-,36,18>)
    n543 = local read "Fr_p"() -> (w1024:fxp<+/-,32,10>)
    n544 = Subtract(x=w1024, y=w1023) -> (x-y=w1021:fxp<+/-,33,11>)
    "fp_tilde" <- w1021
    n545 = local read "fpt_i"() -> (w1015:fxp<+/-,34,18>)
    n546 = Multiply(x="Kp_p", y=w1021) -> (x*y=w1017:fxp<+/-,64,23>)
    n547 = Multiply(x="Kd_p", y=w1019) -> (x*y=w1018:fxp<+/-,64,27>)
    n548 = Absolute Value(x=w1021) -> (abs(x)=w1030:fxp<+,32,10>)
    n549 = Add(x=w1017, y=w1018) -> (x+y=w1013:fxp<+/-,64,28>)
    n550 = Multiply(x="Ki_p", y=w1015) -> (x*y=w1014:fxp<+/-,64,27>)
    n551 = call "Tick Count7"() -> ("Tick Count(uSec)"=w1011:u32)
    n552 = Add(x=w1013, y=w1014) -> (x+y=w1012:fxp<+/-,36,16>)
    n553 = Greater?(x=w1030, y="fp_tolorance") -> (0:w1027:bool)
    n554 = Subtract(x=w1011, y=w1010) -> (x-y=w1009:u32)
    n555 = Divide(x=u32 1000, y=w1009) -> (x/y=→"PID (kHz)":fxp<+/-,20,7>)
    n556 = Select(t=w1012, s=w1027, f=fxp<+,1,1> 0.0) -> (s? t:f=→"Fp_PID":fxp<+/-,36,16>)
  }
  n557 = while "PD position controller_p" {
    stop <- FALSE stop-if-true
    n558 = local read "Drive mode"() -> (w1033:i16)
    n559 = case shown="1" w1033 {
      tunnel: [fxp<+/-,62,19> 0.0 w1036] -> w1032
      frame 0, Default {
        # "Backward"
      }
      frame 1 {
        # "Forward"
        n560 = local read "D_p(mm)"() -> (w1043:fxp<+/-,32,7>)
        n561 = local read "Dp_error_d"() -> (w1035:fxp<+/-,33,8>)
        n562 = local read "Dpr_for"() -> (w1042:fxp<+/-,22,7>)
        n563 = Subtract(x=w1042, y=w1043) -> (x-y=w1041:fxp<+/-,24,8>)
        "Dp_error" <- w1041
        n564 = Multiply(x=w1041, y="Kv_p") -> (x*y=w1038:fxp<+/-,34,16>)
        n565 = Multiply(x=w1035, y="Bv_p") -> (x*y=w1037:fxp<+/-,55,16>)
        n566 = Add(x=w1038, y=w1037) -> (x+y=w1036:fxp<+/-,56,17>)
      }
    }
    "Fr_p" <- w1032
  }
  n567 = while "All switch" {
    stop <- FALSE stop-if-true
    n568 = case shown="True" "Encoder reset" {
      frame False {
        n569 = local write "Encoder reset_p"(FALSE ("Encoder reset_p")) -> ()
        n570 = local write "Encoder reset_y"(FALSE ("Encoder reset_y")) -> ()
      }
      frame True {
        n571 = flat-sequence {
          frame #0 {
            n572 = local write "Encoder reset_p"(TRUE ("Encoder reset_p")) -> ()
          }
          frame #1 {
            n573 = local write "Encoder reset_y"(TRUE ("Encoder reset_y")) -> ()
            n574 = local write "Encoder reset_p"(FALSE ("Encoder reset_p")) -> ()
          }
          frame #2 {
            n575 = local write "Encoder reset_y"(FALSE ("Encoder reset_y")) -> ()
          }
        }
      }
    }
  }
  n576 = while "Derivative" {
    stop <- FALSE stop-if-true
    n577 = local read "Dpr_sin_dd"() -> (w1060:fxp<+/-,35,20>)
    n578 = local read "Stop motor_y"() -> (w1066:bool)
    n579 = local read "Dyr_sin_dd"() -> (w1068:fxp<+/-,35,20>)
    n580 = local read "Dpr_sin_d"() -> (w1062:fxp<+/-,33,15>)
    n581 = local read "Stop motor_p"() -> (w1058:bool)
    n582 = local read "Dyr_sin_d"() -> (w1071:fxp<+/-,33,15>)
    n583 = local read "Dp_error"() -> (w1063:fxp<+/-,22,7>)
    n584 = local read "Dy_error"() -> (w1072:fxp<+/-,22,7>)
    n585 = local read "Dp_dd"() -> (w1061:fxp<+/-,36,25>)
    n586 = local read "Dy_dd"() -> (w1069:fxp<+/-,36,25>)
    n587 = Subtract(x=w1071, y=w1072) -> (x-y=w1070:fxp<+/-,34,16>)
    n588 = Subtract(x=w1068, y=w1069) -> (x-y=w1067:fxp<+/-,41,26>)
    n589 = Subtract(x=w1062, y=w1063) -> (x-y=w1055:fxp<+/-,34,16>)
    n590 = Subtract(x=w1060, y=w1061) -> (x-y=w1059:fxp<+/-,41,26>)
    n591 = Select(t=fxp<+,1,1> 0.0, s=w1066, f=w1070) -> (s? t:f=→"Dy_error_d":fxp<+/-,34,16>)
    n592 = Select(t=fxp<+/-,64,49> 0.0, s=w1066, f=w1067) -> (s? t:f=→"Dy_error_dd":fxp<+/-,64,49>)
    n593 = Select(t=fxp<+,1,1> 0.0, s=w1058, f=w1055) -> (s? t:f=→"Dp_error_d":fxp<+/-,34,16>)
    n594 = Select(t=fxp<+/-,41,26> 0.0, s=w1058, f=w1059) -> (s? t:f=→"Dp_error_dd":fxp<+/-,41,26>)
  }
  n595 = while "ft_d" {
    stop <- FALSE stop-if-true
    n596 = local read "Dy_error_dd"() -> (w1090:fxp<+/-,36,16>)
    n597 = local read "Dp_error_dd"() -> (w1081:fxp<+/-,36,16>)
    n598 = local read "Dy_error_d"() -> (w1092:fxp<+/-,33,8>)
    n599 = local read "Dp_error_d"() -> (w1083:fxp<+/-,33,8>)
    n600 = local read "Kv_p"() -> (w1084:fxp<+/-,22,8>)
    n601 = local read "Bv_p"() -> (w1082:fxp<+/-,22,8>)
    n602 = local read "Kv_y"() -> (w1093:fxp<+/-,22,8>)
    n603 = local read "Bv_y"() -> (w1091:fxp<+/-,22,8>)
    n604 = local read "Force_y"() -> (w1086:fxp<+/-,32,10>)
    n605 = Multiply(x=w1092, y=w1093) -> (x*y=w1088:fxp<+/-,55,16>)
    n606 = Multiply(x=w1090, y=w1091) -> (x*y=w1089:fxp<+/-,58,24>)
    n607 = Multiply(x=w1083, y=w1084) -> (x*y=w1079:fxp<+/-,55,16>)
    n608 = Multiply(x=w1081, y=w1082) -> (x*y=w1080:fxp<+/-,58,24>)
    n609 = local read "Force_p"() -> (w1077:fxp<+/-,32,10>)
    n610 = Add(x=w1088, y=w1089) -> (x+y=w1087:fxp<+/-,63,24>)
    n611 = Add(x=w1079, y=w1080) -> (x+y=w1078:fxp<+/-,63,24>)
    n612 = Subtract(x=w1087, y=w1086) -> (x-y=→"fyt_d":fxp<+/-,63,24>)
    n613 = Subtract(x=w1078, y=w1077) -> (x-y=→"fpt_d":fxp<+/-,63,24>)
  }
  n614 = while "Encoder_y" {
    shift-right: [w1132] -> _
    shift-left: _ -> [w1124]
    shift-right: [w1131] -> _
    shift-left: _ -> [w1123]
    shift-right: [w1122] -> _
    shift-left: _ -> [w1120]
    shift-right: [w1128] -> _
    shift-left: _ -> [w1125]
    shift-right: [w1127] -> _
    shift-left: _ -> [w1126]
    shift-right: [w1121] -> _
    shift-left: _ -> [w1119]
    stop <- FALSE stop-if-true
    w1109 = fxp<+/-,16,1> 0.0244140625  # 2*50/4096
    w1114 = fxp<+/-,20,-5> 0.00048828125  # L/4096
    w1117 = fxp<+/-,20,-5> 0.002499997615814209  # L/800
    w1099 = fxp<+/-,16,1> 0.125  # 2*50/800
    n615 = xnode "FPGA I/O Node"() -> ("Mod7/DIO2"=w1133:bool, "Mod7/DIO3"=w1134:bool)  [unwired: 2 in, 2 out]
    n616 = xnode "FPGA I/O Node"() -> ("Mod7/DIO6"=w1130:bool, "Mod7/DIO7"=w1129:bool)  [unwired: 2 in, 2 out]
    n617 = local read "Encoder reset_y"() -> (w1104:bool)
    n618 = call "encoder_sub.vi"("A_pre"=w1124, "B_pre"=w1123, "Encoder Position_pre"=w1120, "A input"=w1133, "Encoder Position Reset"="Encoder reset_y", "B input"=w1134) -> ("A"=w1132:bool, "B"=w1131:bool, "Encoder Position (Counts)"=w1122:i32)  [unwired: 19 in]
    "Encoder Position_y1" <- w1122
    n619 = call "encoder_sub.vi"("A_pre"=w1125, "B_pre"=w1126, "Encoder Position_pre"=w1119, "A input"=w1130, "Encoder Position Reset"=w1104, "B input"=w1129) -> ("A"=w1128:bool, "B"=w1127:bool, "Encoder Position (Counts)"=w1121:i32)  [unwired: 19 in]
    "Encoder Position_y2" <- w1121
    n620 = local read "Belt_in_y"() -> (w1112:fxp<+/-,6,6>)
    n621 = local read "Belt_in_y"() -> (w1116:fxp<+/-,6,6>)
    n622 = local read "Belt_out_y"() -> (w1110:fxp<+/-,7,7>)
    n623 = Divide(x=w1114, y="Mag. factor_y") -> (x/y=w1113:fxp<+/-,41,13>)
    n624 = local read "Belt_out_y"() -> (w1115:fxp<+/-,7,7>)
    n625 = To Fixed-Point(number=w1121) -> (fixed-point=w1096:fxp<+/-,32,32>)  [unwired: 1 in]
    n626 = local read "Mag. factor_y"() -> (w1108:fxp<+/-,20,3>)
    n627 = To Fixed-Point(number=w1122) -> (fixed-point=w1100:fxp<+/-,32,32>)  [unwired: 1 in]
    n628 = Multiply(x=w1113, y=w1112) -> (x*y=w1111:fxp<+/-,46,18>)
    n629 = Multiply(x=w1117, y=w1116) -> (x*y=w1118:fxp<+/-,26,1>)
    n630 = Divide(x=w1111, y=w1110) -> (x/y=w1098:fxp<+/-,53,18>)
    n631 = Divide(x=w1118, y=w1115) -> (x/y=w1102:fxp<+/-,33,1>)
    n632 = Divide(x=w1109, y=w1108) -> (x/y=w1095:fxp<+/-,32,1>)
    n633 = Multiply(x=w1098, y=w1096) -> (x*y=→"D_y2":fxp<+/-,37,7>)
    n634 = Multiply(x=w1100, y=w1099) -> (x*y=→"rad_y1":fxp<+/-,33,20>)
    n635 = Multiply(x=w1102, y=w1100) -> (x*y=→"D_y1":fxp<+/-,32,7>)
    n636 = Multiply(x=w1096, y=w1095) -> (x*y=→"rad_y2":fxp<+/-,33,20>)
  }
  n637 = while "Omega_y(T method)" {
    shift-right: [w1160] -> _
    shift-left: _ -> [w1161]
    shift-right: [w1147] -> _
    shift-left: _ -> [w1163]
    shift-right: [w1165] -> _
    shift-left: _ -> [w1166]
    shift-right: [w1138] -> _
    shift-left: _ -> [w1139]
    shift-right: [w1136] -> _
    shift-left: _ -> [w1135]
    shift-right: [w1142] -> _
    shift-left: _ -> [w1141]
    stop <- FALSE stop-if-true
    w1154 = fxp<+/-,32,0> 0.3183098859153688  # L/2/pi
    w1159 = fxp<+/-,32,0> 0.3183098859153688  # L/2/pi
    n638 = local read "Encoder Position_y1"() -> (w1160:i32)
    n639 = call "Tick Count2"() -> ("Tick Count(Ticks)"=w1140:u32)
    n640 = local read "Encoder Position_y2"() -> (w1138:i32)
    n641 = call "omega_sub_Encoder_800ppr.vi"("mt0"="mt0_y1", "omega_pre"=w1163, "ticks_m_pre"=w1166, "ticks"=w1140, "count_pre"=w1161, "count"=w1160) -> ("ticks_m"=w1165:u32, "mt"=→"mt_omega_y1":u32, "omega"=w1147:fxp<+/-,36,13>)  [unwired: 3 in]
    "omega_y1 (T)" <- w1147
    n642 = call "omega_sub_Encoder_4096ppr.vi"("mt0"="mt0_y2", "omega_pre"=w1135, "ticks_m_pre"=w1141, "ticks"=w1140, "count_pre"=w1139, "count"=w1138) -> ("ticks_m"=w1142:u32, "mt"=→"mt_omega_y2":u32, "omega"=w1136:fxp<+/-,20,9>)  [unwired: 3 in]
    n643 = local read "Belt_in_y"() -> (w1153:fxp<+/-,6,6>)
    n644 = local read "Mag. factor_y"() -> (w1155:fxp<+/-,20,3>)
    n645 = local read "Belt_out_y"() -> (w1151:fxp<+/-,7,7>)
    n646 = Multiply(x=w1159, y="Belt_in_y") -> (x*y=w1157:fxp<+/-,38,6>)
    n647 = Multiply(x=w1154, y=w1153) -> (x*y=w1152:fxp<+/-,38,6>)
    n648 = Divide(x=w1152, y=w1151) -> (x/y=w1145:fxp<+/-,45,6>)
    n649 = Divide(x=w1157, y="Belt_out_y") -> (x/y=w1148:fxp<+/-,20,1>)
    n650 = Divide(x=w1136, y=w1155) -> (x/y=w1144:fxp<+/-,32,1>)
    "omega_y2 (T)" <- w1144
    n651 = Multiply(x=w1148, y=w1147) -> (x*y=→"Dy1_d (T)":fxp<+/-,36,13>)
    n652 = Multiply(x=w1145, y=w1144) -> (x*y=→"Dy2_d (T)":fxp<+/-,36,13>)
  }
  n653 = xnode "FPGA I/O Node"("error in"=w17, "Mod6/Stop"=TRUE) -> ()  [unwired: 1 in, 2 out]
  n654 = while {
    stop <- FALSE stop-if-true
    n655 = local read "omega_y1 (Mavg)"() -> (w1175:fxp<+/-,36,14>)
    n656 = local read "omega_p1 (Mavg)"() -> (w1179:fxp<+/-,36,14>)
    n657 = local read "Dp1_d (Mavg)"() -> (w1171:fxp<+/-,36,14>)
    n658 = local read "Dy1_d (Mavg)"() -> (w1172:fxp<+/-,36,14>)
    n659 = xnode "Butterworth Filter"("input data"=w1175, "scaled coefficients"="omega_y(Mavg) coeff.") -> ("output data"=→"omega_y (Mavg w. f.)":fxp<+/-,36,18>)  [unwired: 1 in]
    n660 = xnode "Butterworth Filter"("input data"=w1179, "scaled coefficients"="omega_P(Mavg) coeff.") -> ("output data"=→"omega_p (Mavg w. f)":fxp<+/-,36,18>)  [unwired: 1 in]
    n661 = xnode "Butterworth Filter"("input data"=w1172, "scaled coefficients"="Dy_d (Mavg) coeff.") -> ("output data"=→"Dy_d (Mavg w. f.)":fxp<+/-,36,18>)  [unwired: 1 in]
    n662 = xnode "Butterworth Filter"("input data"=w1171, "scaled coefficients"="Dp_d (Mavg) coeff.") -> ("output data"=→"Dp_d (Mavg w. f.)":fxp<+/-,36,18>)  [unwired: 1 in]
  }
